vi "Data Analysis ver2.vi"() -> ()   [LabVIEW 2020]
uses:
  Data converted.ctl
  SignalConversion/FlattenedData.ctl
  Initialization/Param.ctl
  Initialization/ManualCtrl.ctl
  Initialization/DVESetting.ctl
  Initialization/CylinderCalibrNew.ctl
  SignalConversion/DAQChannelOffsets.ctl
  <vilib>/Analysis/Matrix/Datatypes/RealMatrix.ctl
  Data info.ctl
  Tasks/Task/Task.lvclass
  SignalConversion/ScaledData.ctl
  SignalConversion/Measrured TrapXYZ.ctl
  SignalConversion/Data Before Angle Compensation.ctl
  SignalConversion/Angle compensated data.ctl
  SignalConversion/XYZ Signals.ctl
  SignalConversion/Set TrapXYZ.ctl
  SignalConversion/DAQChannelRawData.ctl
  <vilib>/Utility/miscctls.llb/LVFontTypeDef.ctl
  <vilib>/Utility/file.llb/Read From Spreadsheet File (DBL).vi
  <vilib>/Utility/NIReport.llb/NI_report.lvclass
  SignalConversion/SignalConverson.lvlib
  Initialization/FileManagement/FileManagement.lvlib
  BasicVIs/BasicVIs.lvlib
  <vilib>/Analysis/NI_AALBase.lvlib
  <vilib>/Analysis/NI_AALPro.lvlib
  OldDAQtask/HeightFinder/HeightFinder.lvlib
  OldDAQtask/XYcenter/XYcenter.lvlib
  OldDAQtask/Measure angular gains/Measure angular gains.lvlib
  Initialization/Initialization.lvlib
  <vilib>/Analysis/Matrix/NI_Matrix.lvlib
panel:
  in  "stop":bool
  in  "Data Analysis Tab":T1(tab)
  in  "get description from raw data folder?":bool
  in  "Recalculate params":bool
  in  "Fit Method":u16(ring) items=["Reflective 1,3 order", "Symmetric 1,3 order", "1st and 3rd order Func Fit", "7thOrderExpandedWLC"]
  in  "Treat baseline parallel":bool=TRUE
  in  "FitMethod":u16(ring)=1 items=["Fit by two linear functions", "Fit by linear and quadratic "]
  out "%":i32(slide) max=35 scale=0.0..100.0
  in  "Apply new \"config.ini\" file":bool
  in  "configuration file path":path
  out "Trace #":i32(slide) max=35 scale=0.0..7.0
  in  "Raw data root folder":path
  in  "Start conversion":bool
  out "Task #":i32(slide) max=35 scale=0.0..20.0
  in  "Data info":T2 {"params array"."Cylinder Calibr"."ZsignalHeightDependence (1/nm)" format="%.4e"; "params array"."Instrument Calibr"."Psi" format="%#_2f"; "params array"."Manual Control"."Y peizo\n [nm]" step=100.0 scale=0.0..30000.0; "params array"."Manual Control"."AOM0 \nPower" scale=0.0..1.0; "params array"."Manual Control"."X piezo\n [nm]" step=100.0 scale=0.0..30000.0; "params array"."Manual Control"."Rotation Control"."mean freq  [MHz]\ndefault 39.99" min=0.0 step=0.01; "params array"."Manual Control"."Rotation Control"."B amp (0-120)" min=0.0 max=120.0 step=0.1 format="%.1f"; "params array"."Manual Control"."Rotation Control"."A amp (0-120)" min=0.0 max=120.0 step=0.1 format="%.1f"; "params array"."Manual Control"."Rotation Control"."Phase" scale=0.0..360.0; "params array"."Manual Control"."trap height\n [nm]" scale=1000.0..7500.0; "params array"."TaskIDs"."DAQ tasks"."Px taskID" format="%x"; "params array"."TaskIDs"."DAQ tasks"."Py taskID" format="%x"; "params array"."TaskIDs"."DAQ tasks"."Pz taskID" format="%x"; "params array"."TaskIDs"."DAQ tasks"."AOM taskID" format="%x"; "params array"."TaskIDs"."DAQ tasks"."Clock taskID" format="%x"; "params array"."TaskIDs"."DAQ tasks"."AI taskID" format="%x"}
  in  "key words in description":string
  out "Warning message":string
  out "Now converting file:":string
  out "pb1":dbl(slide) scale=0.0..1.0
  out "Descriptions of all traces":string="Trace_0000_Oscilloscope\\description: Initialization and oscilloscope data go here\r\nTrace_0014\\description: good 1\r\nTrace_0019\\description: good 2\r\nTrace_0037\\description: good 3\r\nTrace_0038\\description: good 4 braiding?\r\nTrace_0039\\description: good 4 braiding?\r\nTrace_0044\\description: good 5\r\nTrace_0049\\description: good 6-1\r\nTrace_0050\\description: good 6-2\r\nTrace_0053\\description: good 6-3 cannot achieve last step!!!\r\nTrace_0054\\description: error\r\nTrace_0058\\description: good 6-4 whole\r\nTrace_0059\\description: good 6-5 nucleosome depleted\r\nTrace_0060\\description: good 6-6 nucleosome depleted\r\nTrace_0061\\description: good 6-7 nucleosome depleted\r\nTrace_0062\\description: good 7 non-tc but stretching is good\r\nTrace_0067\\description: good ? 8\r\nTrace_0068\\description: good but break in the middle!\r\nTrace_0069\\description: good but break in the middle!\r\nTrace_0070\\description: braiding?\r\nTrace_0075\\description: good 9 1st multiple winding\r\nTrace_0082\\description: good but break in the middle 10\r\nTrace_0083\\description: good but break in the middle 11\r\nTrace_0086\\description: good weird?\r\nTrace_0092\\description: good only first trace sqeeze the nucleosome out\r\nTrace_0095\\description: good 12 only whole curve got\r\n"
  in  "Data (converted) to import":path
  out "Importing traces..":i32(slide) max=35 scale=0.0..1.0
  in  "Import converted data":bool
  out "Array 2":u32[][](array[colorbox])=[[10162682, 10293497, 10424313, 10555128, 10751479, 10947830, 11143925, 11405812, 11602162, 11864049, 12060399, 12322286, 12453100, 12649451, 12714986, 12780522, 12846058, 12780522, 12714986, 12649451, 12453100, 12322286, 12060399, 11864049, 11602162, 11405812, 11143925, 10947830, 10751479, 10555128, 10424313, 10293497], [10293497, 10424313, 10620664, 10817015, 11013110, 11274996, 11536627, 11864049, 12125679, 12453101, 12714987, 12976872, 13173479, 13369829, 13500900, 13566435, 13631970, 13566435, 13500900, 13369829, 13173479, 12976872, 12714987, 12453101, 12125679, 11864049, 11536627, 11274996, 11013110, 10817015, 10620664, 10424313], [10424313, 10620664, 10817015, 11078645, 11340276, 11667698, 11994864, 12387565, 12714986, 13107943, 13435364, 13762785, 13959390, 14221532, 14352602, 14418137, 14483673, 14418137, 14352602, 14221532, 13959390, 13762785, 13435364, 13107943, 12714986, 12387565, 11994864, 11667698, 11340276, 11078645, 10817015, 10620664], [10555128, 10817015, 11078645, 11405812, 11732978, 12125935, 12518636, 12976872, 13435365, 13828320, 14221532, 14549208, 14811348, 15073744, 15204814, 15270604, 15336139, 15270604, 15204814, 15073744, 14811348, 14549208, 14221532, 13828320, 13435365, 12976872, 12518636, 12125935, 11732978, 11405812, 11078645, 10817015], [10751479, 11013110, 11340276, 11732978, 12191215, 12649451, 13107943, 13631970, 14090461, 14549207, 15008209, 15336139, 15598534, 15795649, 15992510, 16058300, 16058299, 16058300, 15992510, 15795649, 15598534, 15336139, 15008209, 14549207, 14090461, 13631970, 13107943, 12649451, 12191215, 11732978, 11340276, 11013110], [10947830, 11274996, 11667698, 12125935, 12649451, 13173479, 13762785, 14287067, 14811348, 15270604, 15729860, 16058300, 16255669, 16453039, 16519082, 16585128, 16585383, 16585128, 16519082, 16453039, 16255669, 16058300, 15729860, 15270604, 14811348, 14287067, 13762785, 13173479, 12649451, 12125935, 11667698, 11274996], [11143925, 11536627, 11994864, 12518636, 13107943, 13762785, 14352602, 14942674, 15467465, 15926975, 16321204, 16519082, 16717217, 16718490, 16719508, 16720272, 16720527, 16720272, 16719508, 16718490, 16717217, 16519082, 16321204, 15926975, 15467465, 14942674, 14352602, 13762785, 13107943, 12518636, 11994864, 11536627], [11405812, 11864049, 12387565, 12976872, 13631970, 14287067, 14942674, 15532999, 16058300, 16453039, 16651426, 16718998, 16721291, 16657538, 16593531, 16529015, 16463733, 16529015, 16593531, 16657538, 16721291, 16718998, 16651426, 16453039, 16058300, 15532999, 14942674, 14287067, 13631970, 12976872, 12387565, 11864049], [11602162, 12125679, 12714986, 13435365, 14090461, 14811348, 15467465, 16058300, 16453293, 16717726, 16720527, 16657793, 16464244, 16139113, 15879009, 15683677, 15618395, 15683677, 15879009, 16139113, 16464244, 16657793, 16720527, 16717726, 16453293, 16058300, 15467465, 14811348, 14090461, 13435365, 12714986, 12125679], [11864049, 12453101, 13107943, 13828320, 14549207, 15270604, 15926975, 16453039, 16717726, 16721037, 16593531, 16204139, 15683677, 15162449, 14706249, 14445636, 14315074, 14445636, 14706249, 15162449, 15683677, 16204139, 16593531, 16721037, 16717726, 16453039, 15926975, 15270604, 14549207, 13828320, 13107943, 12453101], [12060399, 12714987, 13435364, 14221532, 15008209, 15729860, 16321204, 16651426, 16720527, 16593531, 16139368, 15423318, 14641223, 13858620, 13206067, 12814638, 12684077, 12814638, 13206067, 13858620, 14641223, 15423318, 16139368, 16593531, 16720527, 16651426, 16321204, 15729860, 15008209, 14221532, 13435364, 12714987], [12322286, 12976872, 13762785, 14549208, 15336139, 16058300, 16519082, 16718998, 16657793, 16204139, 15423318, 14445636, 13336629, 12357673, 11574306, 11052061, 10855964, 11052061, 11574306, 12357673, 13336629, 14445636, 15423318, 16204139, 16657793, 16718998, 16519082, 16058300, 15336139, 14549208, 13762785, 12976872], [12453100, 13173479, 13959390, 14811348, 15598534, 16255669, 16717217, 16721291, 16464244, 15683677, 14641223, 13336629, 12031270, 10855964, 9941781, 9353745, 9157904, 9353745, 9941781, 10855964, 12031270, 13336629, 14641223, 15683677, 16464244, 16721291, 16717217, 16255669, 15598534, 14811348, 13959390, 13173479], [12649451, 13369829, 14221532, 15073744, 15795649, 16453039, 16718490, 16657538, 16139113, 15162449, 13858620, 12357673, 10855964, 9549842, 8569868, 7916297, 7720456, 7916297, 8569868, 9549842, 10855964, 12357673, 13858620, 15162449, 16139113, 16657538, 16718490, 16453039, 15795649, 15073744, 14221532, 13369829], [12714986, 13500900, 14352602, 15204814, 15992510, 16519082, 16719508, 16593531, 15879009, 14706249, 13206067, 11574306, 9941781, 8569868, 7524359, 6870789, 6609156, 6870789, 7524359, 8569868, 9941781, 11574306, 13206067, 14706249, 15879009, 16593531, 16719508, 16519082, 15992510, 15204814, 14352602, 13500900], [12780522, 13566435, 14418137, 15270604, 16058300, 16585128, 16720272, 16529015, 15683677, 14445636, 12814638, 11052061, 9353745, 7916297, 6870789, 6216963, 5955586, 6216963, 6870789, 7916297, 9353745, 11052061, 12814638, 14445636, 15683677, 16529015, 16720272, 16585128, 16058300, 15270604, 14418137, 13566435], [12846058, 13631970, 14483673, 15336139, 16058299, 16585383, 16720527, 16463733, 15618395, 14315074, 12684077, 10855964, 9157904, 7720456, 6609156, 5955586, 5759490, 5955586, 6609156, 7720456, 9157904, 10855964, 12684077, 14315074, 15618395, 16463733, 16720527, 16585383, 16058299, 15336139, 14483673, 13631970], [12780522, 13566435, 14418137, 15270604, 16058300, 16585128, 16720272, 16529015, 15683677, 14445636, 12814638, 11052061, 9353745, 7916297, 6870789, 6216963, 5955586, 6216963, 6870789, 7916297, 9353745, 11052061, 12814638, 14445636, 15683677, 16529015, 16720272, 16585128, 16058300, 15270604, 14418137, 13566435], [12714986, 13500900, 14352602, 15204814, 15992510, 16519082, 16719508, 16593531, 15879009, 14706249, 13206067, 11574306, 9941781, 8569868, 7524359, 6870789, 6609156, 6870789, 7524359, 8569868, 9941781, 11574306, 13206067, 14706249, 15879009, 16593531, 16719508, 16519082, 15992510, 15204814, 14352602, 13500900], [12649451, 13369829, 14221532, 15073744, 15795649, 16453039, 16718490, 16657538, 16139113, 15162449, 13858620, 12357673, 10855964, 9549842, 8569868, 7916297, 7720456, 7916297, 8569868, 9549842, 10855964, 12357673, 13858620, 15162449, 16139113, 16657538, 16718490, 16453039, 15795649, 15073744, 14221532, 13369829], [12453100, 13173479, 13959390, 14811348, 15598534, 16255669, 16717217, 16721291, 16464244, 15683677, 14641223, 13336629, 12031270, 10855964, 9941781, 9353745, 9157904, 9353745, 9941781, 10855964, 12031270, 13336629, 14641223, 15683677, 16464244, 16721291, 16717217, 16255669, 15598534, 14811348, 13959390, 13173479], [12322286, 12976872, 13762785, 14549208, 15336139, 16058300, 16519082, 16718998, 16657793, 16204139, 15423318, 14445636, 13336629, 12357673, 11574306, 11052061, 10855964, 11052061, 11574306, 12357673, 13336629, 14445636, 15423318, 16204139, 16657793, 16718998, 16519082, 16058300, 15336139, 14549208, 13762785, 12976872], [12060399, 12714987, 13435364, 14221532, 15008209, 15729860, 16321204, 16651426, 16720527, 16593531, 16139368, 15423318, 14641223, 13858620, 13206067, 12814638, 12684077, 12814638, 13206067, 13858620, 14641223, 15423318, 16139368, 16593531, 16720527, 16651426, 16321204, 15729860, 15008209, 14221532, 13435364, 12714987], [11864049, 12453101, 13107943, 13828320, 14549207, 15270604, 15926975, 16453039, 16717726, 16721037, 16593531, 16204139, 15683677, 15162449, 14706249, 14445636, 14315074, 14445636, 14706249, 15162449, 15683677, 16204139, 16593531, 16721037, 16717726, 16453039, 15926975, 15270604, 14549207, 13828320, 13107943, 12453101], [11602162, 12125679, 12714986, 13435365, 14090461, 14811348, 15467465, 16058300, 16453293, 16717726, 16720527, 16657793, 16464244, 16139113, 15879009, 15683677, 15618395, 15683677, 15879009, 16139113, 16464244, 16657793, 16720527, 16717726, 16453293, 16058300, 15467465, 14811348, 14090461, 13435365, 12714986, 12125679], [11405812, 11864049, 12387565, 12976872, 13631970, 14287067, 14942674, 15532999, 16058300, 16453039, 16651426, 16718998, 16721291, 16657538, 16593531, 16529015, 16463733, 16529015, 16593531, 16657538, 16721291, 16718998, 16651426, 16453039, 16058300, 15532999, 14942674, 14287067, 13631970, 12976872, 12387565, 11864049], [11143925, 11536627, 11994864, 12518636, 13107943, 13762785, 14352602, 14942674, 15467465, 15926975, 16321204, 16519082, 16717217, 16718490, 16719508, 16720272, 16720527, 16720272, 16719508, 16718490, 16717217, 16519082, 16321204, 15926975, 15467465, 14942674, 14352602, 13762785, 13107943, 12518636, 11994864, 11536627], [10947830, 11274996, 11667698, 12125935, 12649451, 13173479, 13762785, 14287067, 14811348, 15270604, 15729860, 16058300, 16255669, 16453039, 16519082, 16585128, 16585383, 16585128, 16519082, 16453039, 16255669, 16058300, 15729860, 15270604, 14811348, 14287067, 13762785, 13173479, 12649451, 12125935, 11667698, 11274996], [10751479, 11013110, 11340276, 11732978, 12191215, 12649451, 13107943, 13631970, 14090461, 14549207, 15008209, 15336139, 15598534, 15795649, 15992510, 16058300, 16058299, 16058300, 15992510, 15795649, 15598534, 15336139, 15008209, 14549207, 14090461, 13631970, 13107943, 12649451, 12191215, 11732978, 11340276, 11013110], [10555128, 10817015, 11078645, 11405812, 11732978, 12125935, 12518636, 12976872, 13435365, 13828320, 14221532, 14549208, 14811348, 15073744, 15204814, 15270604, 15336139, 15270604, 15204814, 15073744, 14811348, 14549208, 14221532, 13828320, 13435365, 12976872, 12518636, 12125935, 11732978, 11405812, 11078645, 10817015], [10424313, 10620664, 10817015, 11078645, 11340276, 11667698, 11994864, 12387565, 12714986, 13107943, 13435364, 13762785, 13959390, 14221532, 14352602, 14418137, 14483673, 14418137, 14352602, 14221532, 13959390, 13762785, 13435364, 13107943, 12714986, 12387565, 11994864, 11667698, 11340276, 11078645, 10817015, 10620664], [10293497, 10424313, 10620664, 10817015, 11013110, 11274996, 11536627, 11864049, 12125679, 12453101, 12714987, 12976872, 13173479, 13369829, 13500900, 13566435, 13631970, 13566435, 13500900, 13369829, 13173479, 12976872, 12714987, 12453101, 12125679, 11864049, 11536627, 11274996, 11013110, 10817015, 10620664, 10424313]]
  out "Fitting result (see block diagram the meanings)":T9
  in  "fit option":u16(ring) items=["Do nothing", "Linear fit", "EWLC fit", "Hat curve fit"]
  out "XY Graph":T10(graph)
  in  "All tasks in tasklist":i32[](listbox)
  in  "Y Axis to plot":i32(ring)=12 items=["V_A' [V]", "V_D' [V]", "V_P'  [V]", "V_S' [V]", "V_L' [V]", "V_R' [V]", "V_sum' [V]", "V_x [V]", "V_y [V]", "V_px' [V]", "V_py' [V]", "V_pz' [V]", "dt [s]", "Vpx_AO [V]", "Vpy_AO [V]", "Vpz_AO [V]", "scan backlog", "LockInPhase", "TrapX [nm]", "TrapY [nm]", "TrapZ [nm]", "V_A [V]", "V_D [V]", "V_P [V]", "V_S [V]", "V_L [V]", "V_R [V]", "V_sum [V]", "V_x [V]", "V_y [V]", "P power [mW]", "S power [mW]", "angle compensated P power [W]", "angle compensated S power [W]", "angle compensated V_L", "angle compensated V_R", "angle compensated V_sum [V]", "angle compensated V_x [V]", "angle compensated V_y [V]", "Psi [rad]", "Laser power before objective[W]", "E_in", "E_out", "Delta E", "X signal", "Y signal", "Z signal", "TrapX (AO) [nm]", "TrapY (AO) [nm]", "TrapZ (AO) [nm]", "Fz [pN]", "Zext [nm]", "Tau [pNnm]", "Turn", "Fx [pN]", "Xext [nm]", "Fy [pN]", "Yext [nm]", "time [s]", "Delta Z signal", "Delta Z bead [nm]", "Z bead [nm]", "Delta TrapZ [nm]", "Delta Xsignal", "X bead [nm]", "Delta Ysignal", "Y bead [nm]", "Stop Condition"]
  in  "X Axis to plot":i32(ring)=12 items=["V_A' [V]", "V_D' [V]", "V_P'  [V]", "V_S' [V]", "V_L' [V]", "V_R' [V]", "V_sum' [V]", "V_x [V]", "V_y [V]", "V_px' [V]", "V_py' [V]", "V_pz' [V]", "dt [s]", "Vpx_AO [V]", "Vpy_AO [V]", "Vpz_AO [V]", "scan backlog", "LockInPhase", "TrapX [nm]", "TrapY [nm]", "TrapZ [nm]", "V_A [V]", "V_D [V]", "V_P [V]", "V_S [V]", "V_L [V]", "V_R [V]", "V_sum [V]", "V_x [V]", "V_y [V]", "P power [mW]", "S power [mW]", "angle compensated P power [W]", "angle compensated S power [W]", "angle compensated V_L", "angle compensated V_R", "angle compensated V_sum [V]", "angle compensated V_x [V]", "angle compensated V_y [V]", "Psi [rad]", "Laser power before objective[W]", "E_in", "E_out", "Delta E", "X signal", "Y signal", "Z signal", "TrapX (AO) [nm]", "TrapY (AO) [nm]", "TrapZ (AO) [nm]", "Fz [pN]", "Zext [nm]", "Tau [pNnm]", "Turn", "Fx [pN]", "Xext [nm]", "Fy [pN]", "Yext [nm]", "time [s]", "Delta Z signal", "Delta Z bead [nm]", "Z bead [nm]", "Delta TrapZ [nm]", "Delta Xsignal", "X bead [nm]", "Delta Ysignal", "Y bead [nm]", "Stop Condition"]
  in  "All traces":i32(listbox)
  in  "Delete trace":bool
  in  "Undo delete":bool
  out "Histogram Graph Y signal (the upmost task)":T11(graph)
  out "mean":dbl format="%0.2f"
  out "s.d.":dbl format="%0.2f"
  out "sigma":dbl format="%0.2f"
  out "center":dbl format="%0.2f"
  in  "Fit":bool
  in  "save to txt":bool
  in  "Save graph":bool
  out "Laser power [W]":dbl format="%0.2f"
  out "Laser power fluctuation [W]":dbl format="%0.2f"
  out "Description":string
  in  "Tab Control":T12(tab)=enum."Settings"
  out "XY Graph for plot 1":T10(graph)
  out "XY Graph for plot 2":T10(graph)
  in  "X Axis to plot 2":i32(ring)=12 items=["V_A' [V]", "V_D' [V]", "V_P'  [V]", "V_S' [V]", "V_L' [V]", "V_R' [V]", "V_sum' [V]", "V_x [V]", "V_y [V]", "V_px' [V]", "V_py' [V]", "V_pz' [V]", "dt [s]", "Vpx_AO [V]", "Vpy_AO [V]", "Vpz_AO [V]", "scan backlog", "LockInPhase", "TrapX [nm]", "TrapY [nm]", "TrapZ [nm]", "V_A [V]", "V_D [V]", "V_P [V]", "V_S [V]", "V_L [V]", "V_R [V]", "V_sum [V]", "V_x [V]", "V_y [V]", "P power [mW]", "S power [mW]", "angle compensated P power [W]", "angle compensated S power [W]", "angle compensated V_L", "angle compensated V_R", "angle compensated V_sum [V]", "angle compensated V_x [V]", "angle compensated V_y [V]", "Psi [rad]", "Laser power before objective[W]", "E_in", "E_out", "Delta E", "X signal", "Y signal", "Z signal", "TrapX (AO) [nm]", "TrapY (AO) [nm]", "TrapZ (AO) [nm]", "Fz [pN]", "Zext [nm]", "Tau [pNnm]", "Turn", "Fx [pN]", "Xext [nm]", "Fy [pN]", "Yext [nm]", "time [s]", "Delta Z signal", "Delta Z bead [nm]", "Z bead [nm]", "Delta TrapZ [nm]", "Delta Xsignal", "X bead [nm]", "Delta Ysignal", "Y bead [nm]", "Stop Condition"]
  in  "Y Axis to plot 2":i32(ring)=12 items=["V_A' [V]", "V_D' [V]", "V_P'  [V]", "V_S' [V]", "V_L' [V]", "V_R' [V]", "V_sum' [V]", "V_x [V]", "V_y [V]", "V_px' [V]", "V_py' [V]", "V_pz' [V]", "dt [s]", "Vpx_AO [V]", "Vpy_AO [V]", "Vpz_AO [V]", "scan backlog", "LockInPhase", "TrapX [nm]", "TrapY [nm]", "TrapZ [nm]", "V_A [V]", "V_D [V]", "V_P [V]", "V_S [V]", "V_L [V]", "V_R [V]", "V_sum [V]", "V_x [V]", "V_y [V]", "P power [mW]", "S power [mW]", "angle compensated P power [W]", "angle compensated S power [W]", "angle compensated V_L", "angle compensated V_R", "angle compensated V_sum [V]", "angle compensated V_x [V]", "angle compensated V_y [V]", "Psi [rad]", "Laser power before objective[W]", "E_in", "E_out", "Delta E", "X signal", "Y signal", "Z signal", "TrapX (AO) [nm]", "TrapY (AO) [nm]", "TrapZ (AO) [nm]", "Fz [pN]", "Zext [nm]", "Tau [pNnm]", "Turn", "Fx [pN]", "Xext [nm]", "Fy [pN]", "Yext [nm]", "time [s]", "Delta Z signal", "Delta Z bead [nm]", "Z bead [nm]", "Delta TrapZ [nm]", "Delta Xsignal", "X bead [nm]", "Delta Ysignal", "Y bead [nm]", "Stop Condition"]
  in  "Plot 1 Options":T14={"Color"=[0, 16711680, 6618880, 16860, 16750610, 4390878, 8388847, 16775234, 5878015, 16740807], "X axis label"="example x", "Y axis label"="example y", "BG color"=16776176, "% axis off"=0.1, "% margin "=2.0, "F: JPEG\nT: PNG"=TRUE, "Font"={"Font Name"="Times New Roman", "Size"=40, "Bold"=TRUE, "Italic"=FALSE, "Underline"=FALSE, "Strikeout"=FALSE, "Color"=0}, "Plot Line Width"=2, "X format str"="%.0f", "Y format str"="%.0f", "axis range"={"Max X scale"=0.0, "Min X scale"=0.0, "Max Y scale"=0.0, "Min Y scale"=0.0}, "auto scale?"=TRUE}
  in  "Plot 2 Options":T14={"Color"=[0, 16711680, 6618880, 16860, 16750610, 4390878, 8388847, 16775234, 5878015, 16740807], "X axis label"="example x", "Y axis label"="example y", "BG color"=16776176, "% axis off"=0.1, "% margin "=2.0, "F: JPEG\nT: PNG"=TRUE, "Font"={"Font Name"="Times New Roman", "Size"=40, "Bold"=TRUE, "Italic"=FALSE, "Underline"=FALSE, "Strikeout"=FALSE, "Color"=0}, "Plot Line Width"=2, "X format str"="%.2f", "Y format str"="%.2f", "axis range"={"Max X scale"=0.0, "Min X scale"=0.0, "Max Y scale"=0.0, "Min Y scale"=0.0}, "auto scale?"=TRUE}
  in  "CreateReport":bool
  in  "Max digit of index":i32=4
  in  "Key words":string="Trace_"
  in  "refresh trace list":bool
  out "array delete order":i32[](array[numeric])
  out "All trace  info":T15(array[cluster]) caption="Folder name                    Description                                                                              Folder index     Key words           Log in finding index"
  in  "path":path caption="path txt saving path"
  out "All descriptions":string="Trace_0000_Oscilloscope\\description: Initialization and oscilloscope data go here\r\nTrace_0014\\description: good 1\r\nTrace_0019\\description: good 2\r\nTrace_0037\\description: good 3\r\nTrace_0038\\description: good 4 braiding?\r\nTrace_0039\\description: good 4 braiding?\r\nTrace_0044\\description: good 5\r\nTrace_0049\\description: good 6-1\r\nTrace_0050\\description: good 6-2\r\nTrace_0053\\description: good 6-3 cannot achieve last step!!!\r\nTrace_0054\\description: error\r\nTrace_0058\\description: good 6-4 whole\r\nTrace_0059\\description: good 6-5 nucleosome depleted\r\nTrace_0060\\description: good 6-6 nucleosome depleted\r\nTrace_0061\\description: good 6-7 nucleosome depleted\r\nTrace_0062\\description: good 7 non-tc but stretching is good\r\nTrace_0067\\description: good ? 8\r\nTrace_0068\\description: good but break in the middle!\r\nTrace_0069\\description: good but break in the middle!\r\nTrace_0070\\description: braiding?\r\nTrace_0075\\description: good 9 1st multiple winding\r\nTrace_0082\\description: good but break in the middle 10\r\nTrace_0083\\description: good but break in the middle 11\r\nTrace_0086\\description: good weird?\r\nTrace_0092\\description: good only first trace sqeeze the nucleosome out\r\nTrace_0095\\description: good 12 only whole curve got\r\n"
  in  "Graph autoname":string[](array[string])
  out "Array of Params out":T3[](array[typedef]) {"Cylinder Calibr"."ZsignalHeightDependence (1/nm)" format="%.4e"; "Instrument Calibr"."Psi" format="%#_2f"; "Manual Control"."Y peizo\n [nm]" step=100.0 scale=0.0..30000.0; "Manual Control"."AOM0 \nPower" scale=0.0..1.0; "Manual Control"."X piezo\n [nm]" step=100.0 scale=0.0..30000.0; "Manual Control"."Rotation Control"."mean freq  [MHz]\ndefault 39.99" min=0.0 step=0.01; "Manual Control"."Rotation Control"."B amp (0-120)" min=0.0 max=120.0 step=0.1 format="%.1f"; "Manual Control"."Rotation Control"."A amp (0-120)" min=0.0 max=120.0 step=0.1 format="%.1f"; "Manual Control"."Rotation Control"."Phase" scale=0.0..360.0; "Manual Control"."trap height\n [nm]" scale=1000.0..7500.0; "TaskIDs"."DAQ tasks"."Px taskID" format="%x"; "TaskIDs"."DAQ tasks"."Py taskID" format="%x"; "TaskIDs"."DAQ tasks"."Pz taskID" format="%x"; "TaskIDs"."DAQ tasks"."AOM taskID" format="%x"; "TaskIDs"."DAQ tasks"."Clock taskID" format="%x"; "TaskIDs"."DAQ tasks"."AI taskID" format="%x"}
  in  "Array of Params const":T3[](array[typedef]) {"Cylinder Calibr"."ZsignalHeightDependence (1/nm)" format="%.4e"; "Instrument Calibr"."Psi" format="%#_2f"; "Manual Control"."Y peizo\n [nm]" step=100.0 scale=0.0..30000.0; "Manual Control"."AOM0 \nPower" scale=0.0..1.0; "Manual Control"."X piezo\n [nm]" step=100.0 scale=0.0..30000.0; "Manual Control"."Rotation Control"."mean freq  [MHz]\ndefault 39.99" min=0.0 step=0.01; "Manual Control"."Rotation Control"."B amp (0-120)" min=0.0 max=120.0 step=0.1 format="%.1f"; "Manual Control"."Rotation Control"."A amp (0-120)" min=0.0 max=120.0 step=0.1 format="%.1f"; "Manual Control"."Rotation Control"."Phase" scale=0.0..360.0; "Manual Control"."trap height\n [nm]" scale=1000.0..7500.0; "TaskIDs"."DAQ tasks"."Px taskID" format="%x"; "TaskIDs"."DAQ tasks"."Py taskID" format="%x"; "TaskIDs"."DAQ tasks"."Pz taskID" format="%x"; "TaskIDs"."DAQ tasks"."AOM taskID" format="%x"; "TaskIDs"."DAQ tasks"."Clock taskID" format="%x"; "TaskIDs"."DAQ tasks"."AI taskID" format="%x"}
  in  "All data after scaling":T16
  in  "All DAQ channels":T22
  in  "empty data info":T2 {"params array"."Cylinder Calibr"."ZsignalHeightDependence (1/nm)" format="%.4e"; "params array"."Instrument Calibr"."Psi" format="%#_2f"; "params array"."Manual Control"."Y peizo\n [nm]" step=100.0 scale=0.0..30000.0; "params array"."Manual Control"."AOM0 \nPower" scale=0.0..1.0; "params array"."Manual Control"."X piezo\n [nm]" step=100.0 scale=0.0..30000.0; "params array"."Manual Control"."Rotation Control"."mean freq  [MHz]\ndefault 39.99" min=0.0 step=0.01; "params array"."Manual Control"."Rotation Control"."B amp (0-120)" min=0.0 max=120.0 step=0.1 format="%.1f"; "params array"."Manual Control"."Rotation Control"."A amp (0-120)" min=0.0 max=120.0 step=0.1 format="%.1f"; "params array"."Manual Control"."Rotation Control"."Phase" scale=0.0..360.0; "params array"."Manual Control"."trap height\n [nm]" scale=1000.0..7500.0; "params array"."TaskIDs"."DAQ tasks"."Px taskID" format="%x"; "params array"."TaskIDs"."DAQ tasks"."Py taskID" format="%x"; "params array"."TaskIDs"."DAQ tasks"."Pz taskID" format="%x"; "params array"."TaskIDs"."DAQ tasks"."AOM taskID" format="%x"; "params array"."TaskIDs"."DAQ tasks"."Clock taskID" format="%x"; "params array"."TaskIDs"."DAQ tasks"."AI taskID" format="%x"}
  out "~All data converted":T23 {"Array of Params"."Cylinder Calibr"."ZsignalHeightDependence (1/nm)" format="%.4e"; "Array of Params"."Instrument Calibr"."Psi" format="%#_2f"; "Array of Params"."Manual Control"."Y peizo\n [nm]" step=100.0 scale=0.0..30000.0; "Array of Params"."Manual Control"."AOM0 \nPower" scale=0.0..1.0; "Array of Params"."Manual Control"."X piezo\n [nm]" step=100.0 scale=0.0..30000.0; "Array of Params"."Manual Control"."Rotation Control"."mean freq  [MHz]\ndefault 39.99" min=0.0 step=0.01; "Array of Params"."Manual Control"."Rotation Control"."B amp (0-120)" min=0.0 max=120.0 step=0.1 format="%.1f"; "Array of Params"."Manual Control"."Rotation Control"."A amp (0-120)" min=0.0 max=120.0 step=0.1 format="%.1f"; "Array of Params"."Manual Control"."Rotation Control"."Phase" scale=0.0..360.0; "Array of Params"."Manual Control"."trap height\n [nm]" scale=1000.0..7500.0; "Array of Params"."TaskIDs"."DAQ tasks"."Px taskID" format="%x"; "Array of Params"."TaskIDs"."DAQ tasks"."Py taskID" format="%x"; "Array of Params"."TaskIDs"."DAQ tasks"."Pz taskID" format="%x"; "Array of Params"."TaskIDs"."DAQ tasks"."AOM taskID" format="%x"; "Array of Params"."TaskIDs"."DAQ tasks"."Clock taskID" format="%x"; "Array of Params"."TaskIDs"."DAQ tasks"."AI taskID" format="%x"}
  out "data deleted":T23 {"Array of Params"."Cylinder Calibr"."ZsignalHeightDependence (1/nm)" format="%.4e"; "Array of Params"."Instrument Calibr"."Psi" format="%#_2f"; "Array of Params"."Manual Control"."Y peizo\n [nm]" step=100.0 scale=0.0..30000.0; "Array of Params"."Manual Control"."AOM0 \nPower" scale=0.0..1.0; "Array of Params"."Manual Control"."X piezo\n [nm]" step=100.0 scale=0.0..30000.0; "Array of Params"."Manual Control"."Rotation Control"."mean freq  [MHz]\ndefault 39.99" min=0.0 step=0.01; "Array of Params"."Manual Control"."Rotation Control"."B amp (0-120)" min=0.0 max=120.0 step=0.1 format="%.1f"; "Array of Params"."Manual Control"."Rotation Control"."A amp (0-120)" min=0.0 max=120.0 step=0.1 format="%.1f"; "Array of Params"."Manual Control"."Rotation Control"."Phase" scale=0.0..360.0; "Array of Params"."Manual Control"."trap height\n [nm]" scale=1000.0..7500.0; "Array of Params"."TaskIDs"."DAQ tasks"."Px taskID" format="%x"; "Array of Params"."TaskIDs"."DAQ tasks"."Py taskID" format="%x"; "Array of Params"."TaskIDs"."DAQ tasks"."Pz taskID" format="%x"; "Array of Params"."TaskIDs"."DAQ tasks"."AOM taskID" format="%x"; "Array of Params"."TaskIDs"."DAQ tasks"."Clock taskID" format="%x"; "Array of Params"."TaskIDs"."DAQ tasks"."AI taskID" format="%x"}
  in  "data of tasks in single trace":T25
  in  "empty data converted":T23 {"Array of Params"."Cylinder Calibr"."ZsignalHeightDependence (1/nm)" format="%.4e"; "Array of Params"."Instrument Calibr"."Psi" format="%#_2f"; "Array of Params"."Manual Control"."Y peizo\n [nm]" step=100.0 scale=0.0..30000.0; "Array of Params"."Manual Control"."AOM0 \nPower" scale=0.0..1.0; "Array of Params"."Manual Control"."X piezo\n [nm]" step=100.0 scale=0.0..30000.0; "Array of Params"."Manual Control"."Rotation Control"."mean freq  [MHz]\ndefault 39.99" min=0.0 step=0.01; "Array of Params"."Manual Control"."Rotation Control"."B amp (0-120)" min=0.0 max=120.0 step=0.1 format="%.1f"; "Array of Params"."Manual Control"."Rotation Control"."A amp (0-120)" min=0.0 max=120.0 step=0.1 format="%.1f"; "Array of Params"."Manual Control"."Rotation Control"."Phase" scale=0.0..360.0; "Array of Params"."Manual Control"."trap height\n [nm]" scale=1000.0..7500.0; "Array of Params"."TaskIDs"."DAQ tasks"."Px taskID" format="%x"; "Array of Params"."TaskIDs"."DAQ tasks"."Py taskID" format="%x"; "Array of Params"."TaskIDs"."DAQ tasks"."Pz taskID" format="%x"; "Array of Params"."TaskIDs"."DAQ tasks"."AOM taskID" format="%x"; "Array of Params"."TaskIDs"."DAQ tasks"."Clock taskID" format="%x"; "Array of Params"."TaskIDs"."DAQ tasks"."AI taskID" format="%x"}
  # "Tools"
  # "Statistics:"
  # "Channels in page 2:"
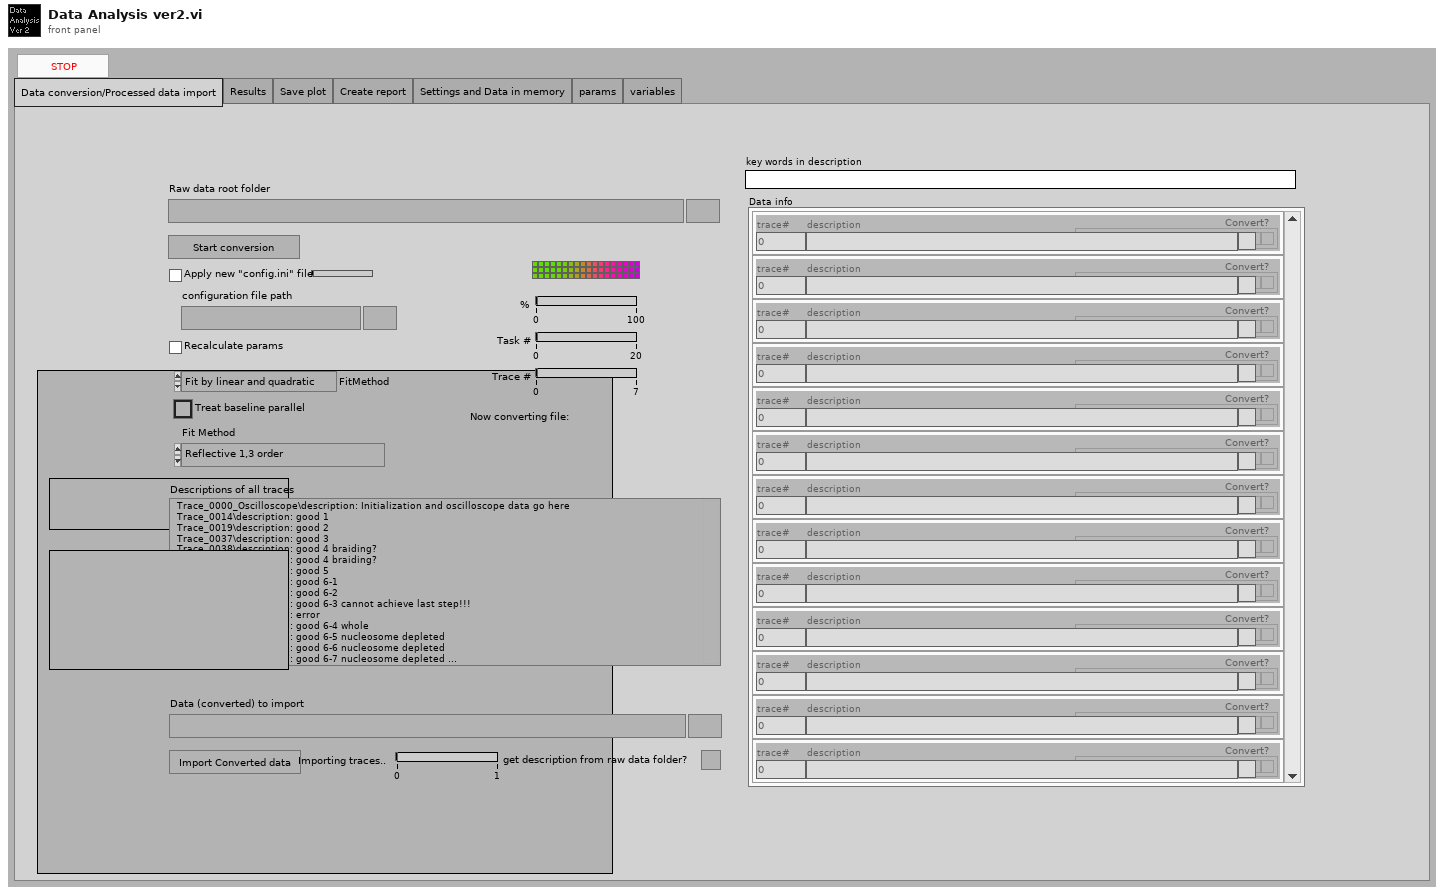
[diagram p1: front panel]
types:
  T1 = enum32{"Data conversion/Processed data import", "Results", "Save plot", "Create report", "Settings and Data in memory", "params", "variables"}
  T2 = typedef "Data info.ctl" = cluster{"trace#":i32, cluster{"index":i32, "File path":path, "File name":string}[], "description":string, "Convert?":bool, "params array":T3[], "Array":refnum<class "Task.lvclass">[]}[]
  T3 = typedef "Initialization.lvlib/Param.ctl" = cluster{"TaskIDs":cluster{"DAQ tasks":cluster{"Px taskID":u32, "Py taskID":u32, "Pz taskID":u32, "AOM taskID":u32, "Clock taskID":u32, "AI taskID":u32}, "DVEHandle":refnum<file>}, "Manual Control":T4, "Piezo Calibr":cluster{"Px2Vx(AO)":dbl, "Py2Vy(AO)":dbl, "Pz2Vz(AO)":dbl, "Min Px":dbl, "Min Py":dbl, "Min Pz":dbl, "Max Px":dbl, "Max Py":dbl, "Max Pz":dbl, "Vx0 (V)":dbl, "Vy0 (V)":dbl, "Vz0 (V)":dbl}, "Instrument Calibr":cluster{"Angular compensation coeffs":dbl[][], "TetherCenter":cluster{"TrapX_AO 0 [nm]":dbl, "TrapY_AO 0 [nm]":dbl, "TrapZ_AO 0 [nm]":dbl}, "XYZsignal baseline":cluster{"Xsignal0":dbl, "Ysignal0":dbl, "Zsignal0":dbl, "Zsig slope":dbl, "Z bead0":dbl}, "S and P to Vs0":cluster{"Vs0/P":dbl, "Vs0/S":dbl}, "Psi":dbl, "ePS:eRL drift correlation":cluster{"Interc P":dbl, "Slope P":dbl, "Interc S":dbl, "Slope S":dbl}, "Current piezo volt AO":cluster{"Vpx_AO [V]":dbl, "Vpy_AO [V]":dbl, "Vpz_AO [V]":dbl}}, "Cylinder Calibr":T6, "DAQParams":cluster{"Buffer size":dbl, "Scanning rate":dbl, "Average":dbl, "Sampling rate":dbl, "set dt":dbl}, "DAQ channel offsets":T7, "Z bead polynomial coeffs":dbl[], "Skip button ref":refnum<vi>, "z bead lookup table":cluster{"z signal":dbl[], "z bead":dbl[]}, "SP->power Matrix":T8, "Ms2p":T8, "Mp2s":T8, "Polynomial coeff V_px,y,z 2 position (nm)":dbl[][]}
  T4 = typedef "Initialization.lvlib/ManualCtrl.ctl" = cluster{"Rotation Control":T5, "X piezo\n [nm]":dbl, "Y peizo\n [nm]":dbl, "trap height\n [nm]":dbl, "AOM0 \nPower":dbl}
  T5 = typedef "Initialization.lvlib/DVESetting.ctl" = cluster{"Phase":dbl, "A amp (0-120)":dbl, "B amp (0-120)":dbl, "mean freq  [MHz]\ndefault 39.99":dbl, "freq difference [Hz]":dbl, "Enable A":bool, "Enable B":bool}
  T6 = typedef "Initialization.lvlib/CylinderCalibrNew.ctl" = cluster{"ZStiff":dbl, "Zsens":dbl, "AngStiff":dbl, "XStiff":dbl, "Xsens":dbl, "MaxEllip":dbl, "YStiff":dbl, "Ysens":dbl, "FocalShift":dbl, "Sfz":dbl, "1/Sz":dbl, "Stau":dbl, "Sfx":dbl, "1/Sx":dbl, "1/Sang":dbl, "Sfy":dbl, "1/Sy":dbl, "1/focal":dbl, "ZsignalHeightDependence (1/nm)":dbl}
  T7 = typedef "SignalConverson.lvlib/DAQChannelOffsets.ctl" = cluster{"A0 [V]":dbl, "D0 [V]":dbl, "P0  [V]":dbl, "S0 [V]":dbl, "L0 [V]":dbl, "R0 [V]":dbl, "Vpx0 [V]":dbl, "Vpy0 [V]":dbl, "Vpz0 [V]":dbl, "Vsum0 [V]":dbl, "Vpx_AO0 [V]":dbl, "Vpy_AO0 [V]":dbl, "Vpz_AO0 [V]":dbl}
  T8 = typedef "NI_Matrix.lvlib/RealMatrix.ctl" = dbl[][]
  T9 = cluster{"coeff 0":dbl, "coeff 1":dbl, "coeff 2":dbl, "coeff 3":dbl}
  T10 = cluster{"Processed data":dbl[], "Processed data":dbl[]}[]
  T11 = cluster{"X Values":dbl[], "Best Gaussian Fit":dbl[]}[]
  T12 = enum32{"Plot 1 (=plot in \"Reults\" tab)", "Page 2", "Settings"}
  T13 = typedef "LVFontTypeDef.ctl" = cluster{"Font Name":string, "Size":u16, "Bold":bool, "Italic":bool, "Underline":bool, "Strikeout":bool, "Color":u32}
  T14 = cluster{"Color":u32[], "X axis label":string, "Y axis label":string, "BG color":u32, "% axis off":dbl, "% margin ":dbl, "F: JPEG\nT: PNG":bool, "Font":T13, "Plot Line Width":u8, "X format str":string, "Y format str":string, "axis range":cluster{"Max X scale":dbl, "Min X scale":dbl, "Max Y scale":dbl, "Min Y scale":dbl}, "auto scale?":bool}
  T15 = cluster{"Folder index":i32, "Date modefied":i32, "Folder name":string, "Description":string, "Key words":string, "Log in Finding index":string}[]
  T16 = typedef "SignalConverson.lvlib/ScaledData.ctl" = cluster{"Measured TrapXYZ":T17, "Data before ang comp":T18, "Data after angle compensation":T19, "X,Y,Z signal":T20, "Set TrapXYZ":T21}
  T17 = typedef "SignalConverson.lvlib/Measrured TrapXYZ.ctl" = cluster{"TrapX [nm]":dbl, "TrapY [nm]":dbl, "TrapZ [nm]":dbl}
  T18 = typedef "SignalConverson.lvlib/Data Before Angle Compensation.ctl" = cluster{"V_A [V]":dbl, "V_D [V]":dbl, "V_P [V]":dbl, "V_S [V]":dbl, "V_L [V]":dbl, "V_R [V]":dbl, "V_sum [V]":dbl, "V_x [V]":dbl, "V_y [V]":dbl, "P power [mW]":dbl, "S power [mW]":dbl}
  T19 = typedef "SignalConverson.lvlib/Angle compensated data.ctl" = cluster{"angle compensated P power [W]":dbl, "angle compensated S power [W]":dbl, "angle compensated V_L":dbl, "angle compensated V_R":dbl, "angle compensated V_sum [V]":dbl, "angle compensated V_x [V]":dbl, "angle compensated V_y [V]":dbl, "Psi [rad]":dbl, "Laser power before objective[W]":dbl, "E_in":dbl, "E_out":dbl, "Delta E":dbl}
  T20 = typedef "SignalConverson.lvlib/XYZ Signals.ctl" = cluster{"X signal":dbl, "Y signal":dbl, "Z signal":dbl}
  T21 = typedef "SignalConverson.lvlib/Set TrapXYZ.ctl" = cluster{"TrapX (AO) [nm]":dbl, "TrapY (AO) [nm]":dbl, "TrapZ (AO) [nm]":dbl}
  T22 = typedef "SignalConverson.lvlib/DAQChannelRawData.ctl" = cluster{"V_A' [V]":dbl, "V_D' [V]":dbl, "V_P'  [V]":dbl, "V_S' [V]":dbl, "V_L' [V]":dbl, "V_R' [V]":dbl, "V_sum' [V]":dbl, "V_x [V]":dbl, "V_y [V]":dbl, "V_px' [V]":dbl, "V_py' [V]":dbl, "V_pz' [V]":dbl, "dt [s]":dbl, "Vpx_AO [V]":dbl, "Vpy_AO [V]":dbl, "Vpz_AO [V]":dbl, "scan backlog":u32, "LockInPhase":dbl}
  T23 = typedef "Data converted.ctl" = cluster{cluster{"trace (folder) name":string, "task (file) name":string, "processed data":T24[]}[], "tasklist (name)":string[], "trace name":string, "description":string, "Array of Params":T3[]}[]
  T24 = typedef "SignalConverson.lvlib/FlattenedData.ctl" = cluster{"V_A' [V]":dbl, "V_D' [V]":dbl, "V_P'  [V]":dbl, "V_S' [V]":dbl, "V_L' [V]":dbl, "V_R' [V]":dbl, "V_sum' [V]":dbl, "V_x [V]":dbl, "V_y [V]":dbl, "V_px' [V]":dbl, "V_py' [V]":dbl, "V_pz' [V]":dbl, "dt [s]":dbl, "Vpx_AO [V]":dbl, "Vpy_AO [V]":dbl, "Vpz_AO [V]":dbl, "scan backlog":dbl, "LockInPhase":dbl, "TrapX [nm]":dbl, "TrapY [nm]":dbl, "TrapZ [nm]":dbl, "V_A [V]":dbl, "V_D [V]":dbl, "V_P [V]":dbl, "V_S [V]":dbl, "V_L [V]":dbl, "V_R [V]":dbl, "V_sum [V]":dbl, "V_x [V]":dbl, "V_y [V]":dbl, "P power [mW]":dbl, "S power [mW]":dbl, "angle compensated P power [W]":dbl, "angle compensated S power [W]":dbl, "angle compensated V_L":dbl, "angle compensated V_R":dbl, "angle compensated V_sum [V]":dbl, "angle compensated V_x [V]":dbl, "angle compensated V_y [V]":dbl, "Psi [rad]":dbl, "Laser power before objective[W]":dbl, "E_in":dbl, "E_out":dbl, "Delta E":dbl, "X signal":dbl, "Y signal":dbl, "Z signal":dbl, "TrapX (AO) [nm]":dbl, "TrapY (AO) [nm]":dbl, "TrapZ (AO) [nm]":dbl, "Fz [pN]":dbl, "Zext [nm]":dbl, "Tau [pNnm]":dbl, "Turn":dbl, "Fx [pN]":dbl, "Xext [nm]":dbl, "Fy [pN]":dbl, "Yext [nm]":dbl, "time [s]":dbl, "Delta Z signal":dbl, "Delta Z bead [nm]":dbl, "Z bead [nm]":dbl, "Delta TrapZ [nm]":dbl, "Delta Xsignal":dbl, "X bead [nm]":dbl, "Delta Ysignal":dbl, "Y bead [nm]":dbl, "Stop Condition":dbl}
  T25 = cluster{"folder name":string, "file name":string, "Processed data":T24[]}
  T26 = enum16{"open", "replace", "create", "open or create", "replace or create", "replace or create with confirmation"}
  T27 = cluster{cluster{"trace (folder) name":string, "task (file) name":string, "processed data":T24[]}[], "tasklist (name)":string[], "trace name":string, "description":string, "Array of Params":T3[]}
  T28 = cluster{"trace#":i32, cluster{"index":i32, "File path":path, "File name":string}[], "description":string, "Convert?":bool, "params array":T3[], "Array":refnum<class "Task.lvclass">[]}
  T29 = cluster{cluster{"trace (folder) name":string, "task (file) name":string, "processed data":T24[]}[], "tasklist (name)":string[], "trace name":string, "description":string, "Array of Params":T3[]}[]
  T30 = cluster{"index":i32, "File path":path, "File name":string}[]
  T31 = typedef "SignalConverson.lvlib/Physical Quantitites.ctl" = cluster{"Fz [pN]":dbl, "Zext [nm]":dbl, "Tau [pNnm]":dbl, "Turn":dbl, "Fx [pN]":dbl, "Xext [nm]":dbl, "Fy [pN]":dbl, "Yext [nm]":dbl, "time [s]":dbl, "Delta Z signal":dbl, "Delta Z bead [nm]":dbl, "Z bead [nm]":dbl, "Delta TrapZ [nm]":dbl, "Delta Xsignal":dbl, "X bead [nm]":dbl, "Delta Ysignal":dbl, "Y bead [nm]":dbl, "Stop Condition":dbl}
  T32 = cluster{"index cross = max-1":bool, "index cross = max-2":bool, "index cross = 0":bool, "index cross = 1":bool, "Exceeds max iter":bool, "no solution 2rd order polyn ":bool}
  T33 = cluster{"trace (folder) name":string, "task (file) name":string, "processed data":T24[]}[]
  T34 = cluster{"p":dbl, "l0":dbl, "k0":dbl, "residue":dbl}
  T35 = typedef "Initialization.lvlib/FileManagement.lvlib/Folder information.ctl" = cluster{"Folder index":i32, "Date modefied":i32, "Folder name":string, "Description":string, "Key words":string, "Log in Finding index":string}[]
  T36 = cluster{"Folder index":i32, "dup file":path, string}
  T37 = cluster{"Folder index":i32, "appended path":path, string}
  T38 = cluster{"Folder index":i32, "appended path":path, string}[]
  T39 = cluster{"trace (folder) name":string, "task (file) name":string, "processed data":T24[]}
  T40 = cluster{"X Values":dbl[], "Histogram: h(x)":i32[]}
  T41 = cluster{"X Values":dbl[], "Best Gaussian Fit":dbl[]}
  T42 = typedef "LVPointDoubleTypeDef.ctl" = cluster{"Cursor X":dbl, "Cursor Y":dbl}
  T43 = cluster{string, string, "Flattened data 1D array":T24[]}
  T44 = cluster{cluster{string, string, "Flattened data 1D array":T24[]}[], string[], string, string, "Array of Params const":T3[]}
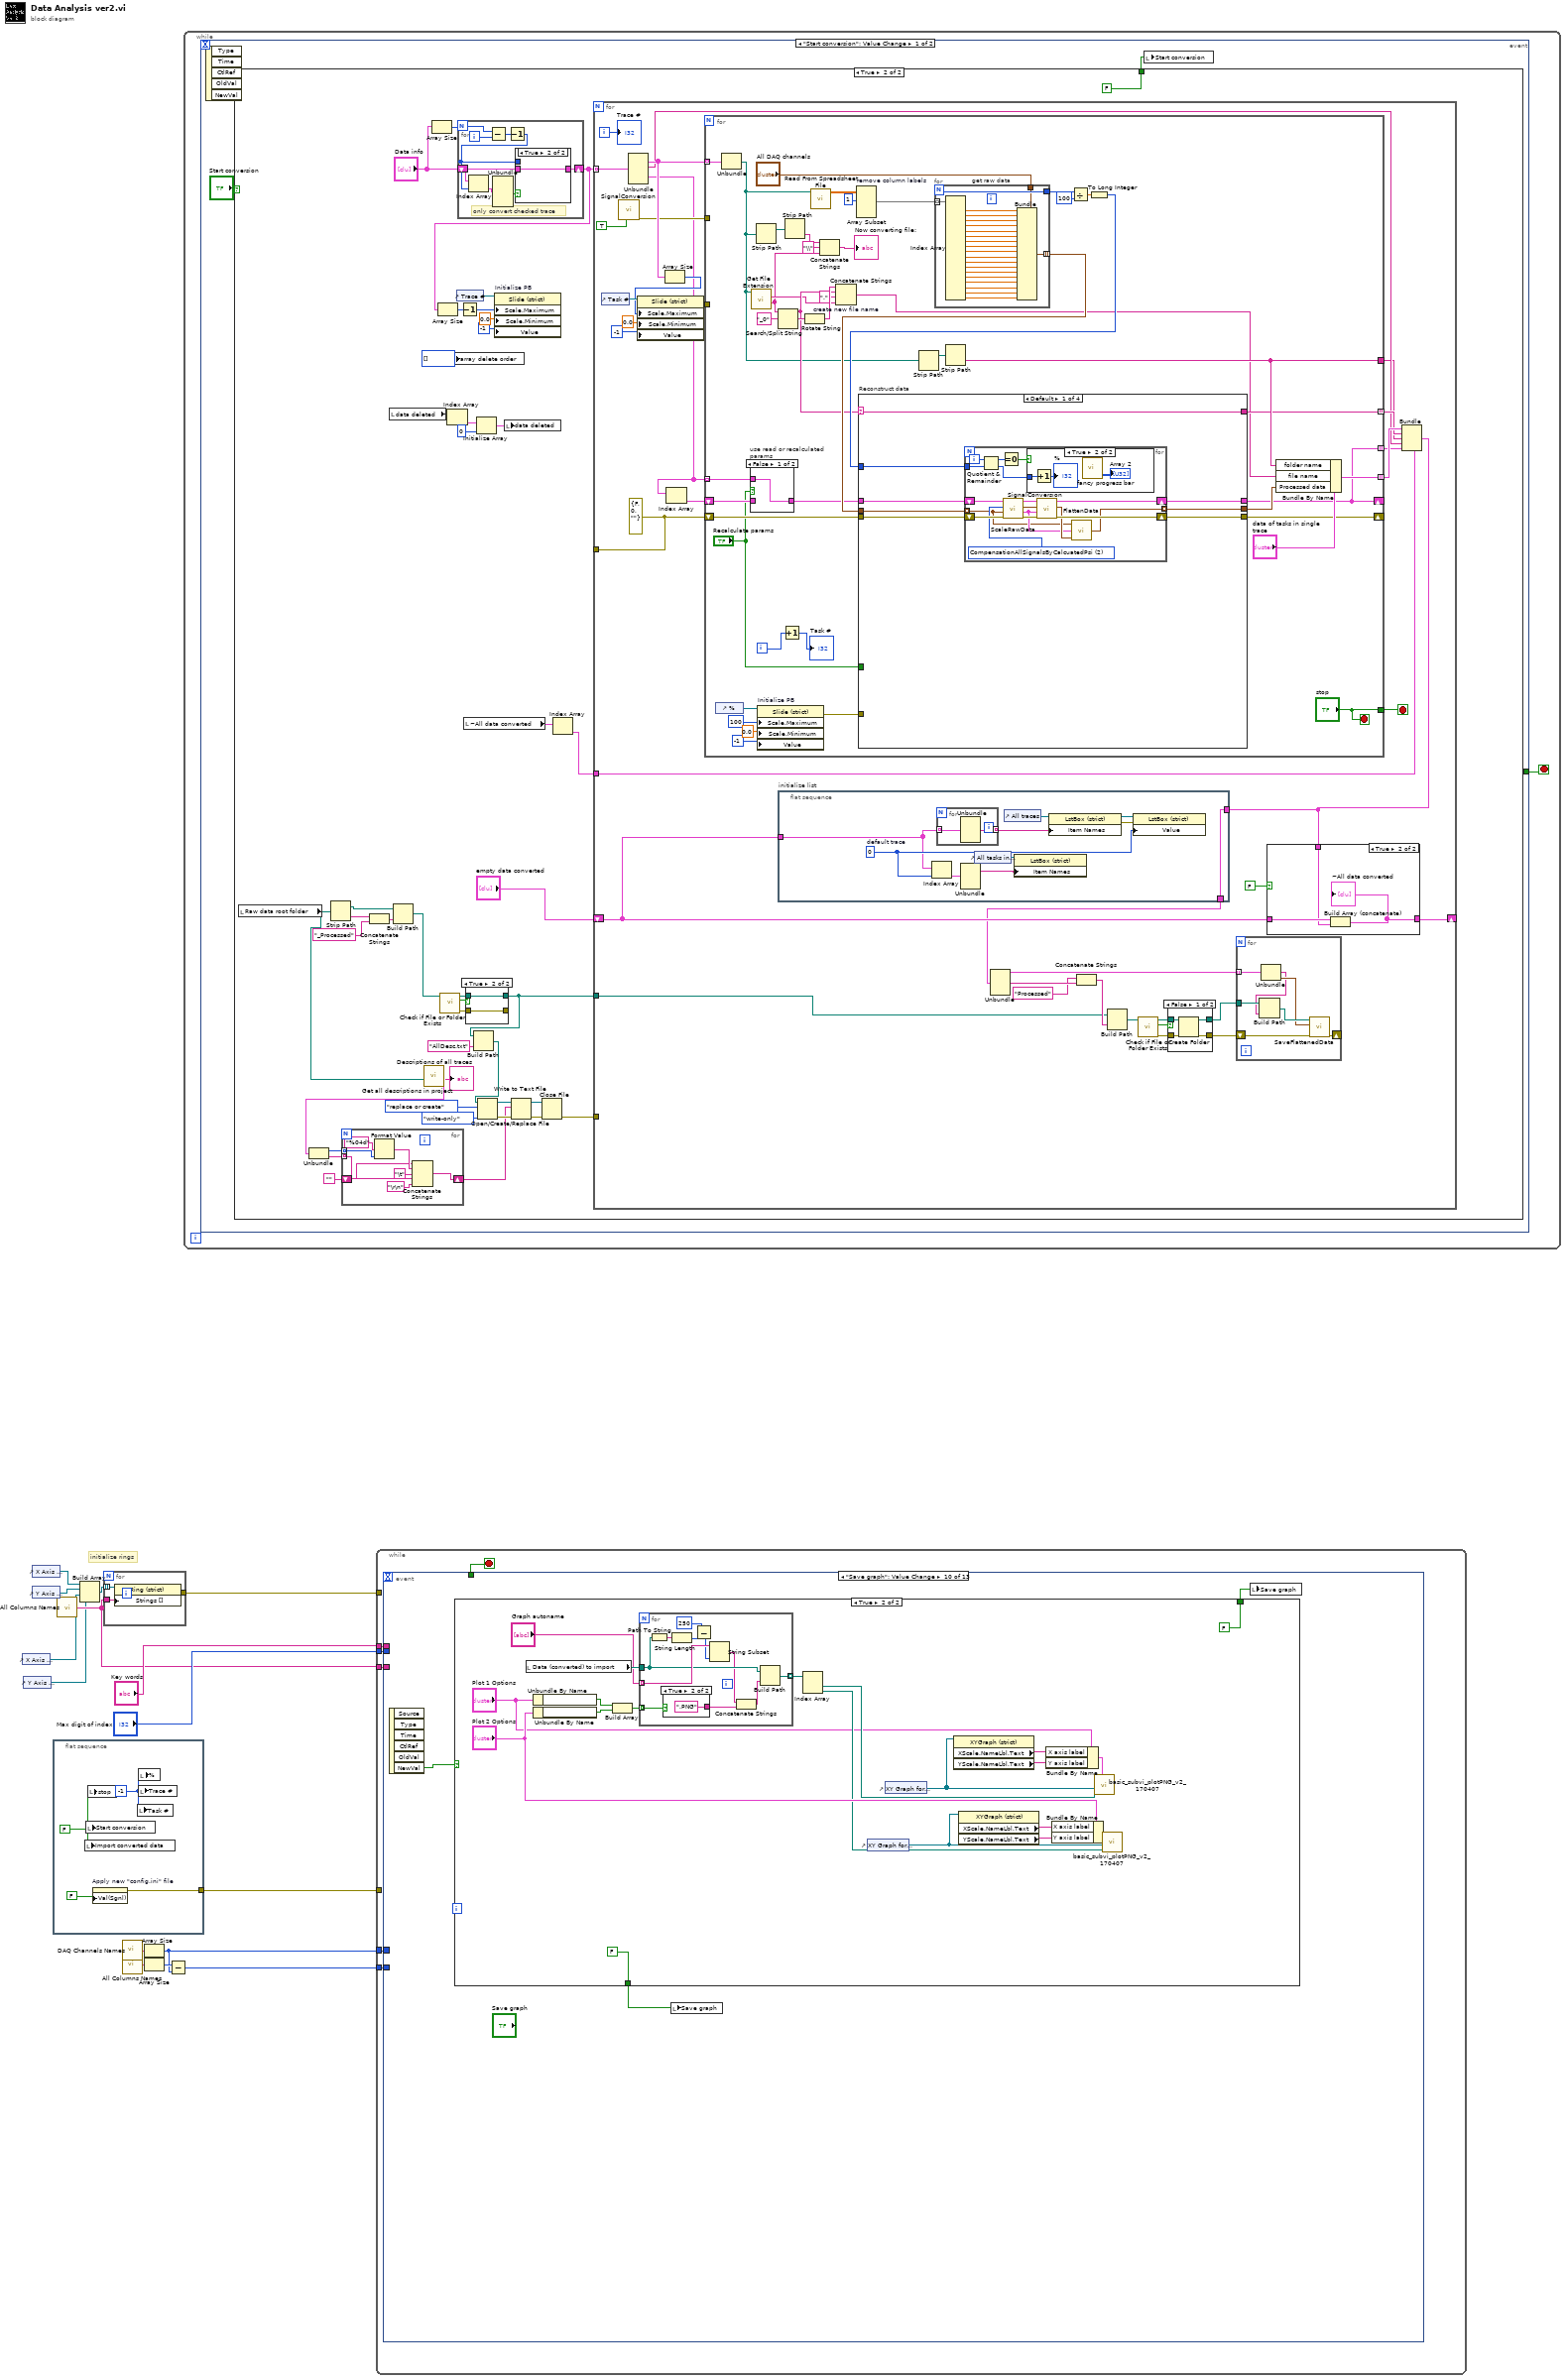
[diagram p0: block diagram]
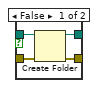
[diagram p3: hidden frame]
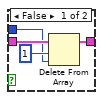
[diagram p4: hidden frame]
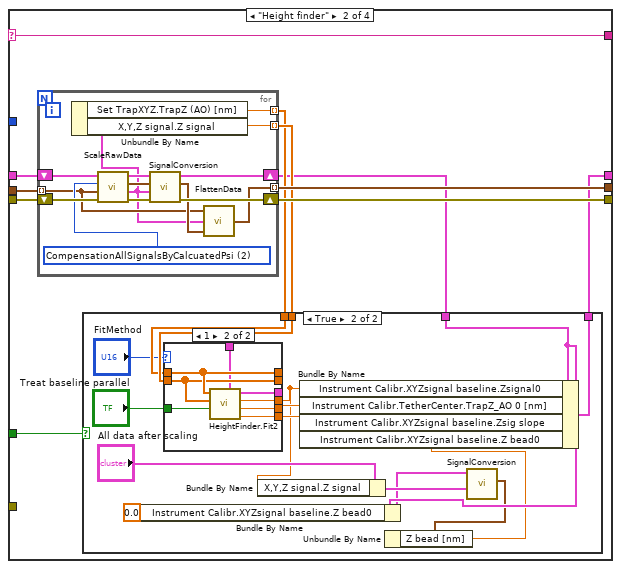
[diagram p9: hidden frame]
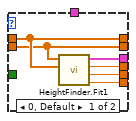
[diagram p11: hidden frame]
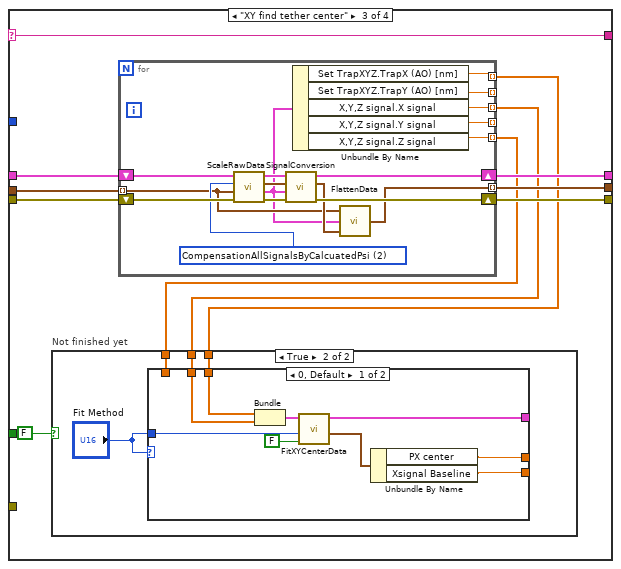
[diagram p12: hidden frame]
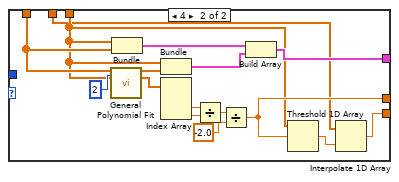
[diagram p14: hidden frame]
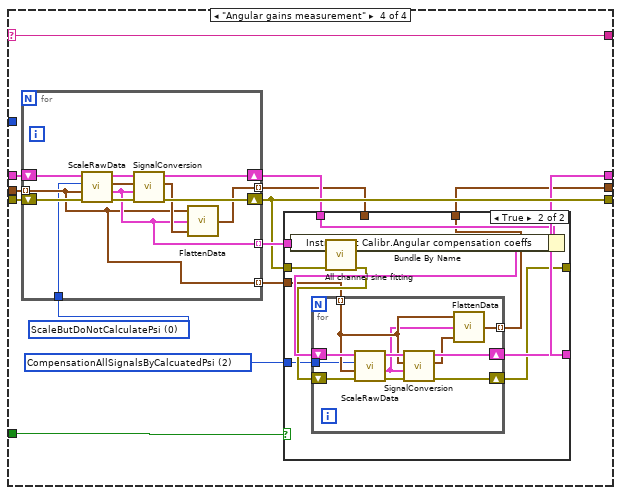
[diagram p15: hidden frame]
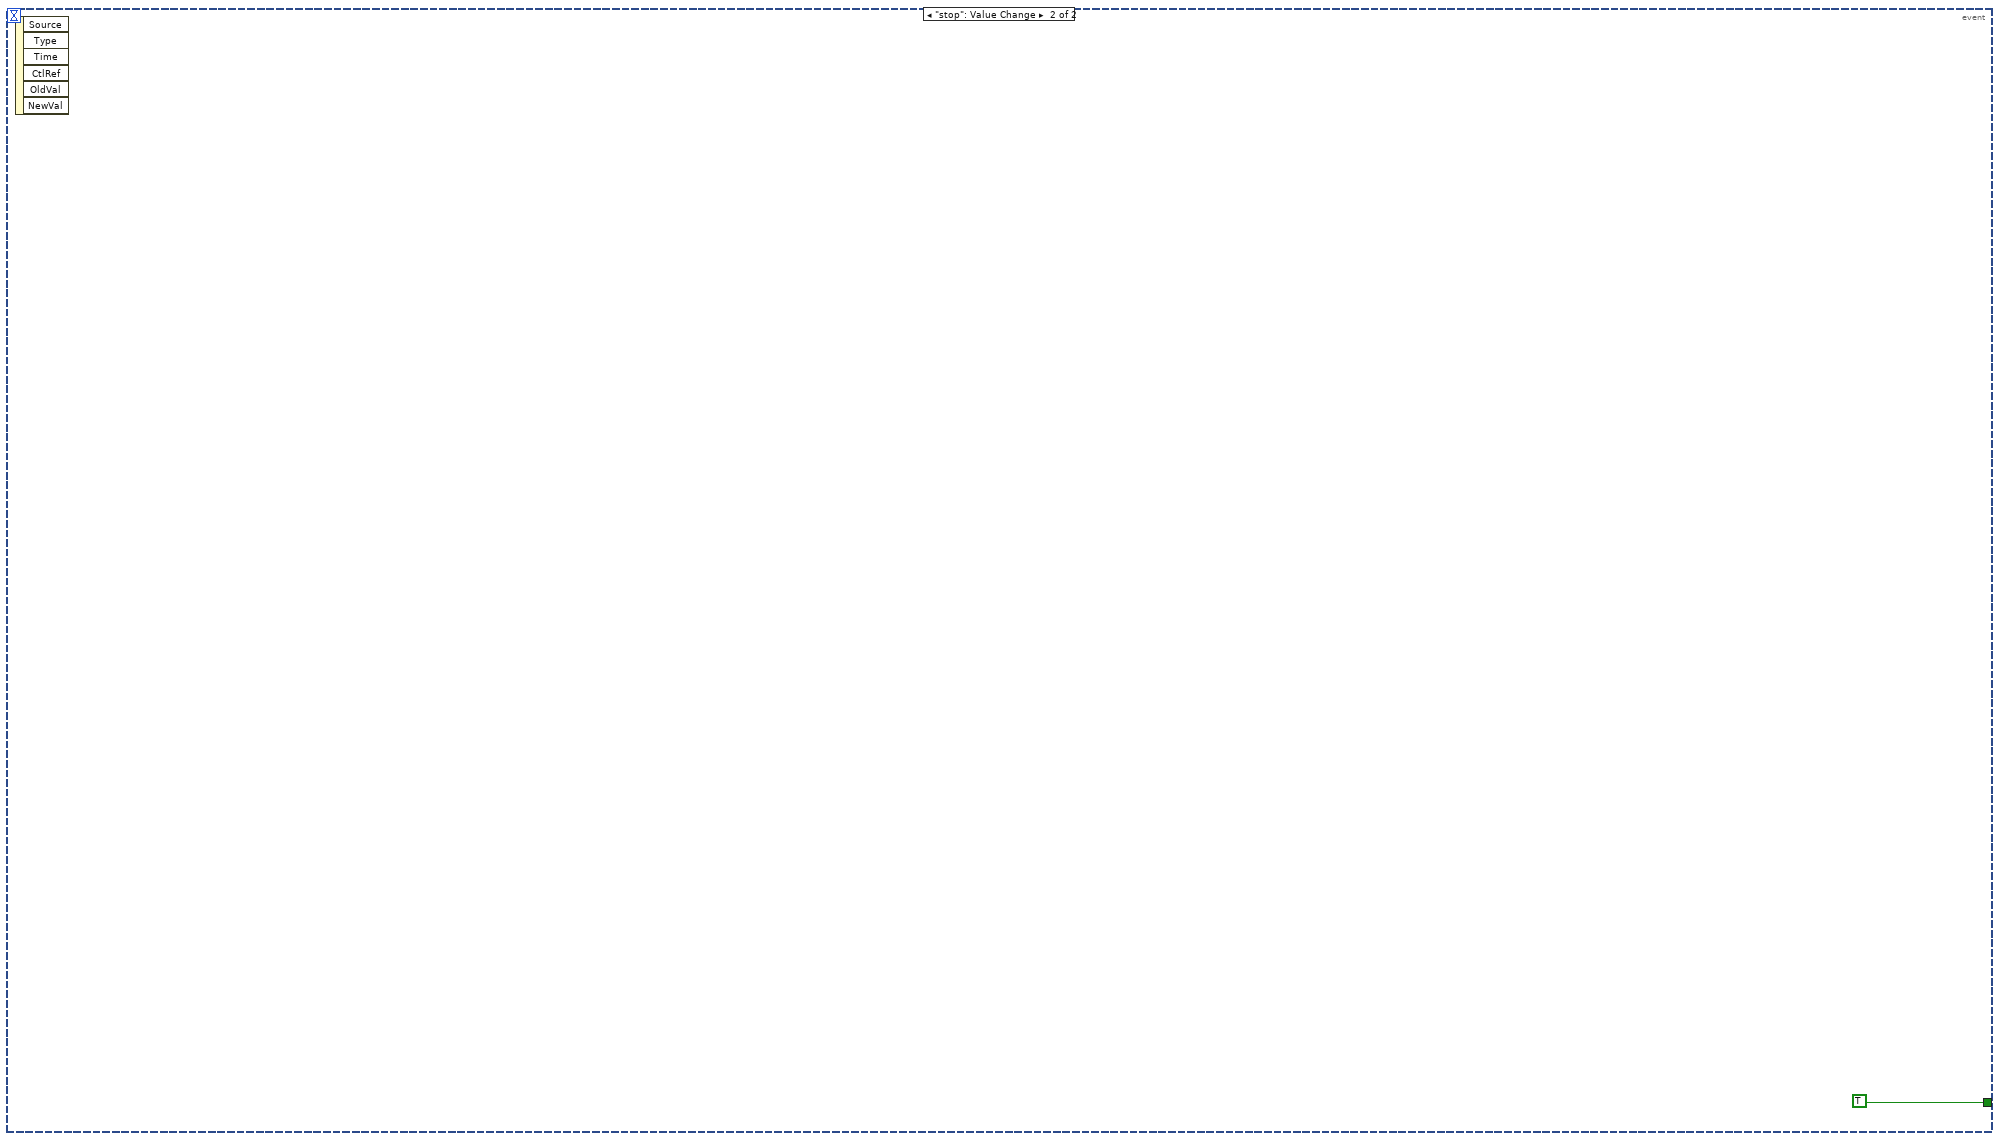
[diagram p17: hidden frame]
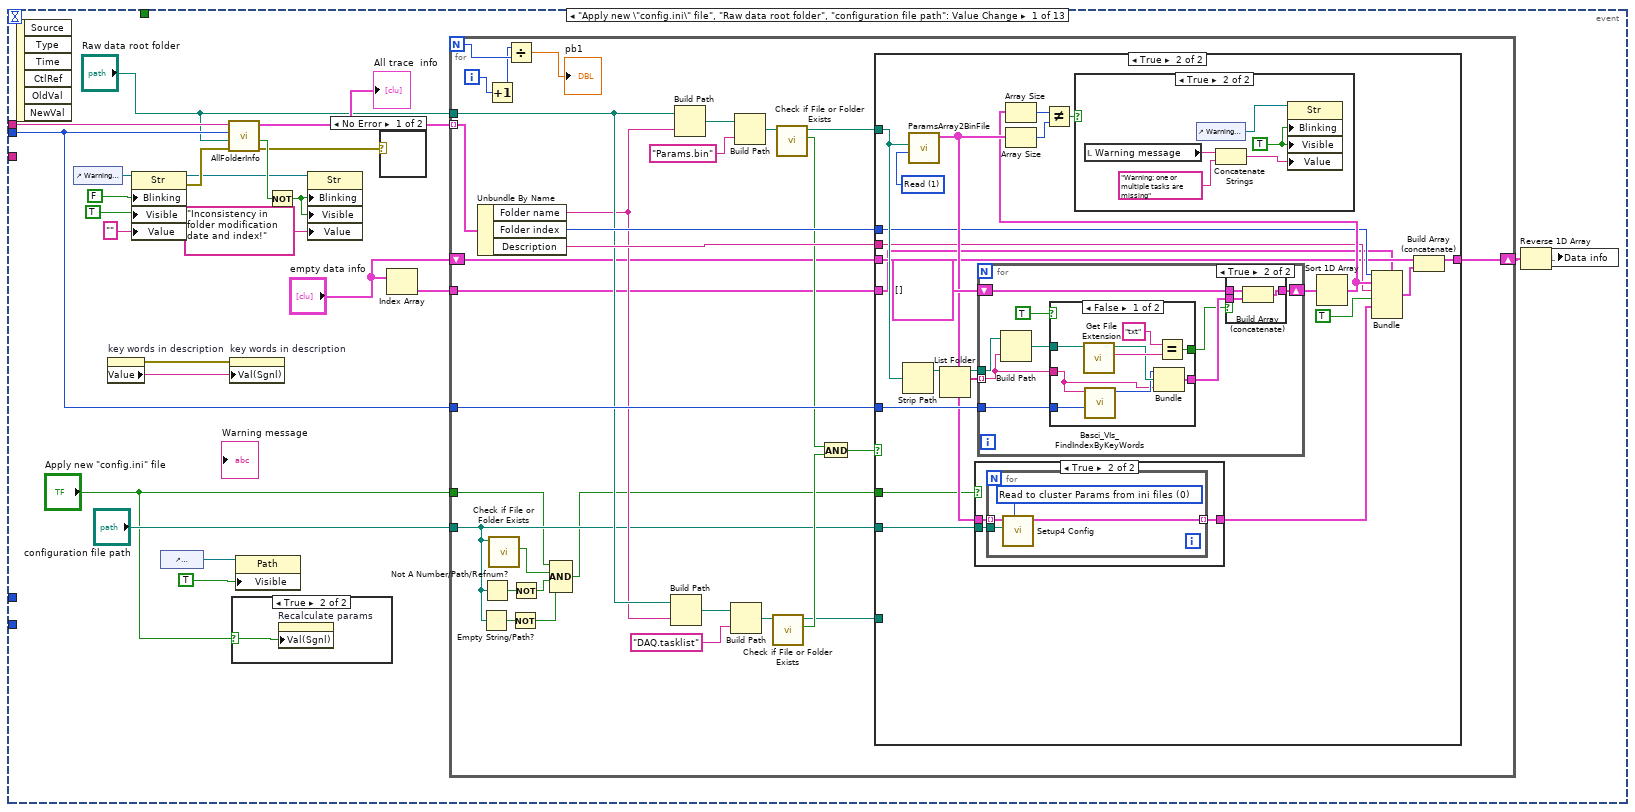
[diagram p18: hidden frame]
diagram:
  # "initialize rings"
  n1 = control-ref of="X Axis to plot 2"() -> (w2:refnum<vi>)
  n2 = control-ref of="Y Axis to plot 2"() -> (w1:refnum<vi>)
  n3 = control-ref of="X Axis to plot"() -> (w6:refnum<vi>)
  n4 = control-ref of="Y Axis to plot"() -> (w7:refnum<vi>)
  n5 = flat-sequence {
    tunnel: [w18] -> w15
    frame #0 {
      w19 = -1 ("%")
      w17 = FALSE ("Start conversion")
      n6 = local write "Import converted data"(w17) -> ()
      n7 = local write "Start conversion"(w17) -> ()
      n8 = local write "stop"(w17) -> ()
      n9 = property on="Apply new \"config.ini\" file" class="Bool (strict)"("Val(Sgnl)"=FALSE ("Blinking")) -> (error out=w18:errorcluster)  [unwired: 2 in, 1 out]
      n10 = local write "Task #"(w19) -> ()
      n11 = local write "Trace #"(w19) -> ()
      n12 = local write "%"(w19) -> ()
    }
  }
  n13 = call "All Columns Names.vi"() -> ("All column names"=w3:string[])
  n14 = Build Array(w6, w7, w2, w1) -> (w5:refnum<vi>[])
  n15 = for {
    tunnel: w5 -> [w22] mode=indexing
    tunnel: w3 -> [w21]
    tunnel: [w20] -> w4
    n16 = property class="Ring (strict)"(reference=w22, "Strings []"=w21) -> (error out=w20:errorcluster)  [unwired: 1 in, 1 out]
  }
  n17 = call "DAQ Channels Names.vi"() -> ("DAQ channel names (string)"=w12:string[])  [unwired: 7 in]
  n18 = call "All Columns Names.vi"() -> ("All column names"=w11:string[])
  n19 = Array Size(array=w12) -> (size(s)=w9:i32)
  n20 = Array Size(array=w11) -> (size(s)=w10:i32)
  n21 = Subtract(x=w10, y=w9) -> (x-y=w8:i32)
  n22 = while {
    stop <- w23 stop-if-true
    n23 = event shown="[0] \"Start conversion\": Value Change" {
      selector: _ -> [_ _]
      dyn-events: _ -> [_ _]
      timeout: _ -> [_ _]
      tunnel: [_ TRUE] -> w23
      event "Start conversion": Value Change {
        n24 = event-data() -> ()  [unwired: 1 in, 5 out]
        n25 = case shown="True" "Start conversion" {
          tunnel: [_ FALSE ("start conversion 2")] -> w25
          frame False {
          }
          frame True {
            n26 = local read "Raw data root folder"() -> (w42:path)
            n27 = Strip Path(path=w42) -> (stripped path=w46:path, name=w48:string)
            n28 = Concatenate Strings(w48, "_Processed" ("string")) -> (w49:string)
            n29 = local read "data deleted"() -> (w57:T23)
            n30 = Build Path(base path=w46, name or relative path=w49) -> (appended path=w50:path)
            n31 = call "Get all descriptions in project.vi"("Folder Path"=w42) -> ("All descriptions"=→"Descriptions of all traces":string, "Descriptions and trace index"=w35:cluster{i32[], string[]})  [unwired: 7 in]
            n32 = Unbundle(w35) -> (w34:i32[], w33:string[])
            n33 = for {
              tunnel: w34 -> [w75] mode=indexing
              tunnel: w33 -> [w72] mode=indexing
              shift-right: [w69] -> w31
              shift-left: "" -> [w68]
              n34 = Format Value(format string="%04d" ("string (\"\")"), value (0)=w75) -> (output string=w73:string)  [unwired: 1 in]
              n35 = Concatenate Strings(w68, w73, "\t", w72, "\r\n") -> (w69:string)
            }
            n36 = Array Size(array="Data info") -> (size(s)=w65:i32)
            n37 = call <vilib>:"Check if File or Folder Exists.vi"("path"=w50) -> ("error out"=w45:errorcluster, "file or folder exists?"=w43:bool, "dup path"=w44:path)  [unwired: 8 in]
            n38 = Index Array(array=w57) -> (element=w56:T27)  [unwired: 1 in]
            n39 = local write "array delete order"(i32[] [] ("array delete order")) -> ()
            n40 = control-ref of="Trace #"() -> (w63:refnum<vi>)
            n41 = for {
              N: w65 -> [w88]
              shift-right: [w89] -> w59
              shift-left: "Data info" -> [w85]
              i -> [w87]
              # "only convert checked trace"
              n42 = Subtract(x=w88, y=w87) -> (x-y=w86:i32)
              n43 = Decrement(x=w86) -> (x-1=w82:i32)
              n44 = Index Array(array=w85, index=w82) -> (element=w84:T28)
              n45 = Unbundle(w84) -> ("Convert?"=w83:bool)  [unwired: 5 out]
              n46 = case shown="True" w83 {
                tunnel: w85 -> [w93 w94]
                tunnel: [w92 w94] -> w89
                tunnel: w82 -> [w90 _]
                frame False {
                  n47 = Delete From Array(array=w93, length=1, index=w90) -> (array with subset deleted=w92:T2)  [unwired: 1 out]
                }
                frame True {
                }
              }
            }
            n48 = Array Size(array=w59) -> (size(s)=w64:i32)
            n49 = Decrement(x=w64) -> (x-1=w60:i32)
            n50 = local read "~All data converted"() -> (w53:T23)
            n51 = case shown="True" w43 {
              tunnel: [w79 w81] -> w41
              tunnel: [w78 w80] -> _
              tunnel: w45 -> [w77 w80]
              tunnel: w44 -> [w76 w81]
              frame False {
                n52 = Create Folder(path (use dialog)=w76, error in=w77) -> (created path=w79:path, error out=w78:errorcluster)  [unwired: 1 in, 1 out]
              }
              frame True {
              }
            }
            n53 = Build Path(base path=w41, name or relative path="AllDesc.txt") -> (appended path=w39:path)
            n54 = Initialize Array(w56, 0 ("dimension size")) -> (w54:T29)
            n55 = Open/Create/Replace File(file path (use dialog)=w39, operation (0:open)=T26."replace or create", access (0:read/write)=enum16{"read/write", "read-only", "write-only"}."write-only") -> (refnum out=w29:refnum<file>, error out=w36:errorcluster)  [unwired: 3 in, 1 out]
            n56 = property on="Initialize PB" class="Slide (strict)"(reference=w63, "Scale.Maximum"=w60, "Scale.Minimum"=0.0 ("Scale.Range:Minimum"), "Value"=-1 ("标尺.范围:最小值")) -> ()  [unwired: 1 in, 2 out]
            n57 = local write "data deleted"(w54) -> ()
            n58 = Write to Text File(file (use dialog)=w29, text=w31, error in=w36) -> (refnum out=w27:refnum<file>, error out=w28:errorcluster)  [unwired: 1 in, 1 out]
            n59 = Close File(refnum=w27, error in=w28) -> (error out=w26:errorcluster)  [unwired: 1 out]
            n60 = Index Array(array=w53) -> (element=w52:T27)  [unwired: 1 in]
            n61 = for {
              tunnel: w59 -> [w124] mode=indexing
              tunnel: w52 -> [w112]
              shift-right: [w111] -> _
              shift-left: "empty data converted" -> [w110]
              tunnel: [w109] -> _
              tunnel: w41 -> [w98]
              tunnel: w26 -> [_]
              i -> [w127]
              stop <- w125 stop-if-true
              w109 = errorcluster {"status"=FALSE, "code"=0, "source"=""} ("error out")
              n62 = control-ref of="Task #"() -> (w130:refnum<vi>)
              n63 = call "SignalConversion.vi"("Reinitialize time? (F)"=TRUE) -> ("error out"=w121:errorcluster)  [unwired: 6 in, 4 out]
              n64 = Unbundle(w124) -> (w122:T30, "description"=w117:string, "params array"=w116:T3[])  [unwired: 3 out]
              n65 = Array Size(array=w122) -> (size(s)=w123:i32)
              n66 = property on="属性节点" class="Slide (strict)"(reference=w130, "Scale.Maximum"=w123, "Scale.Minimum"=0.0 ("Scale.Range:Minimum"), "Value"=-1 ("标尺.范围:最小值")) -> (error out=w126:errorcluster)  [unwired: 1 in, 1 out]
              n67 = Index Array(array=w116) -> (element=w115:T3)  [unwired: 1 in]
              n68 = for {
                tunnel: w122 -> [w197] mode=indexing
                tunnel: [w196] -> w113
                tunnel: [w182] -> w118 mode=indexing
                tunnel: w126 -> [_]
                tunnel: ["stop"] -> w125
                tunnel: w116 -> [w180] mode=indexing
                tunnel: w121 -> [_]
                tunnel: [w193] -> w119 mode=indexing
                shift-right: [w177] -> _
                shift-left: w115 -> [w179]
                shift-right: [w184] -> _
                shift-left: w109 -> [w185]
                tunnel: [w177] -> w114 mode=indexing
                i -> [w167]
                stop <- "stop" stop-if-true
                n69 = control-ref of="%"() -> (w201:refnum<vi>)
                n70 = Unbundle(w197) -> ("File path"=w165:path)  [unwired: 2 out]
                n71 = case "use read or recalculated params" shown="False" "Recalculate params" {
                  tunnel: w180 -> [w204 _]
                  tunnel: [w204 w205] -> w178
                  tunnel: w179 -> [_ w205]
                  frame False {
                  }
                  frame True {
                  }
                }
                n72 = call <vilib>:"Get File Extension.vi"("file"=w165) -> ("filename without extension"=w163:string, "lowercase file extension"=w170:string)  [unwired: 6 in, 3 out]
                n73 = Strip Path(path=w165) -> (stripped path=w164:path)  [unwired: 1 out]
                n74 = property on="Initialize PB" class="Slide (strict)"(reference=w201, "Scale.Maximum"=100 ("y"), "Scale.Minimum"=0.0 ("Scale.Range:Minimum"), "Value"=-1 ("标尺.范围:最小值")) -> (error out=w181:errorcluster)  [unwired: 1 in, 1 out]
                n75 = Search/Split String(string=w163, search string/char (-)="_0") -> (substring before match=w171:string, match + rest of string=w173:string)  [unwired: 1 in, 1 out]
                n76 = Increment(x=w167) -> (x+1=→"Task #":i32)
                n77 = Strip Path(path=w164) -> (name=w161:string)  [unwired: 1 out]
                n78 = Rotate String(1:w173) -> (0:w172:string)
                n79 = call-poly <vilib>:"Read From Spreadsheet File.vi"("file path (dialog if empty)"=w165) -> ("all rows"=w194:dbl[][])  [unwired: 6 in, 4 out]
                n80 = Concatenate Strings(w161, "\\" ("string"), w163) -> (→"Now converting file:":string)
                n81 = Concatenate Strings "create new file name"(w172, w171, "." ("string"), w170) -> (w169:string)
                n82 = Array Subset "remove column labels"(array=w194, index (row)=1 ("index")) -> (w191:dbl[][])  [unwired: 3 in]
                n83 = Strip Path(path=w165) -> (stripped path=w202:path)  [unwired: 1 out]
                n84 = for "get raw data" {
                  N -> [w398]
                  tunnel: w191 -> [w401] mode=indexing
                  tunnel: [w399] -> w186 mode=indexing
                  tunnel: [w398] -> w189
                  tunnel: "All DAQ channels" -> [w397]
                  n85 = Index Array(array=w401) -> (element #1=w402:dbl, element #2=w403:dbl, element #3=w404:dbl, element #4=w405:dbl, element #5=w406:dbl, element #6=w407:dbl, element #7=w408:dbl, element #8=w409:dbl, element #9=w410:dbl, element #10=w411:dbl, element #11=w412:dbl, element #12=w413:dbl, element #13=w414:dbl, element #14=w415:dbl, element #15=w416:dbl, element #16=w417:dbl, element #17=w418:dbl, element #18=w400:dbl)  [unwired: 18 in]
                  n86 = Bundle(cluster=w397, "V_A' [V]"=w402, "V_D' [V]"=w403, "V_P'  [V]"=w404, "V_S' [V]"=w405, "V_L' [V]"=w406, "V_R' [V]"=w407, "V_sum' [V]"=w408, "V_x [V]"=w409, "V_y [V]"=w410, "V_px' [V]"=w411, "V_py' [V]"=w412, "V_pz' [V]"=w413, "dt [s]"=w414, "Vpx_AO [V]"=w415, "Vpy_AO [V]"=w416, "Vpz_AO [V]"=w417, "scan backlog"=w418, "LockInPhase"=w400) -> (w399:T22)
                }
                n87 = Strip Path(path=w202) -> (name=w196:string)  [unwired: 1 out]
                n88 = Divide(x=w189, y=100) -> (x/y=w190:dbl)
                n89 = To Long Integer(number=w190) -> (32bit integer=w187:i32)
                n90 = case "Reconstruct data" shown="Default" w171 {
                  selector: w171 -> [w206 w239 w293 w356]
                  tunnel: w187 -> [w213 _ _ _]
                  tunnel: w186 -> [w212 w244 w299 w359]
                  tunnel: [w211 w234 w298 w350] -> w177
                  tunnel: [w210 w243 w297 w353] -> w184
                  tunnel: w185 -> [w209 w242 w296 w358]
                  tunnel: w178 -> [w208 w241 w295 w357]
                  tunnel: [w207 w240 w294 w348] -> w183
                  tunnel: [w206 w239 w293 w356] -> w182
                  tunnel: w181 -> [_ _ _ _]
                  tunnel: "Recalculate params" -> [_ w236 _ w354]
                  frame Default {
                    n91 = for {
                      shift-right: [w226] -> w210
                      shift-left: w209 -> [w227]
                      shift-right: [w225] -> w211
                      shift-left: w208 -> [w230]
                      tunnel: w213 -> [w224]
                      tunnel: [w218] -> w207 mode=indexing
                      tunnel: w212 -> [w214] mode=indexing
                      i -> [w223]
                      w215 = 2 items=["ScaleButDoNotCalculatePsi", "CalculatePsi, ButDoNotCompensate", "CompensationAllSignalsByCalcuatedPsi", "DoNotScale(ReadRawVoltageSignals)"] ("Scale Option")
                      n92 = Quotient & Remainder(x=w223, y=w224) -> (x-y*floor(x/y)=w222:i32, floor(x/y)=w220:i32)
                      n93 = Equal To 0?(x=w222) -> (x = 0?=w221:bool)
                      n94 = call "ScaleRawData.vi"("error in (no error)"=w227, "All DAQ channels"=w214, "Scale Option"=w215, "Params in"=w230) -> ("error out"=w228:errorcluster, "Scaled data"=w216:T16, "All DAQ channels out"=w219:T22, "Params out"=w229:T3)  [unwired: 1 in]
                      n95 = case shown="True" w221 {
                        tunnel: w220 -> [_ w233]
                        frame False {
                        }
                        frame True {
                          n96 = Increment(x=w233) -> (x+1=→"%":i32)
                          n97 = call "fancy progress bar.vi"() -> ("Array 2"=→"Array 2":u32[][])  [unwired: 1 in, 1 out]
                        }
                      }
                      n98 = call "SignalConversion.vi"("error in (no error)"=w228, "All data after scaling"=w216, "All DAQ channels"=w219, "Params in"=w229) -> ("error out"=w226:errorcluster, "Physical Quantities cluster out"=w217:T31, "Params out"=w225:T3)  [unwired: 3 in, 2 out]
                      n99 = call "FlattenData.vi"("Physical Quantities"=w217, "All data after scaling"=w216, "All DAQ channels"=w214) -> ("Flattened data"=w218:T24)  [unwired: 2 in]
                    }
                  }
                  frame "Height finder" {
                    n100 = for {
                      shift-right: [w284] -> w243
                      shift-left: w242 -> [w285]
                      shift-right: [w283] -> w235
                      shift-left: w241 -> [w288]
                      tunnel: [w281] -> w240 mode=indexing
                      tunnel: w244 -> [w278] mode=indexing
                      tunnel: [w276] -> w238 mode=indexing
                      tunnel: [w275] -> w237 mode=indexing
                      w279 = 2 items=["ScaleButDoNotCalculatePsi", "CalculatePsi, ButDoNotCompensate", "CompensationAllSignalsByCalcuatedPsi", "DoNotScale(ReadRawVoltageSignals)"] ("Scale Option")
                      n101 = call "ScaleRawData.vi"("error in (no error)"=w285, "All DAQ channels"=w278, "Scale Option"=w279, "Params in"=w288) -> ("error out"=w286:errorcluster, "Scaled data"=w277:T16, "All DAQ channels out"=w282:T22, "Params out"=w287:T3)  [unwired: 1 in]
                      n102 = Unbundle By Name(w277) -> ("Set TrapXYZ.TrapZ (AO) [nm]"=w275:dbl, "X,Y,Z signal.Z signal"=w276:dbl)
                      n103 = call "SignalConversion.vi"("error in (no error)"=w286, "All data after scaling"=w277, "All DAQ channels"=w282, "Params in"=w287) -> ("error out"=w284:errorcluster, "Physical Quantities cluster out"=w280:T31, "Params out"=w283:T3)  [unwired: 3 in, 2 out]
                      n104 = call "FlattenData.vi"("Physical Quantities"=w280, "All data after scaling"=w277, "All DAQ channels"=w278) -> ("Flattened data"=w281:T24)  [unwired: 2 in]
                    }
                    n105 = case shown="True" w236 {
                      tunnel: w238 -> [_ w260]
                      tunnel: w237 -> [_ w259]
                      tunnel: w235 -> [w245 w249]
                      tunnel: [w245 w250] -> w234
                      frame False {
                      }
                      frame True {
                        n106 = Bundle By Name(cluster=w249, "Instrument Calibr.XYZsignal baseline.Z bead0"=0.0) -> (w248:T3)
                        n107 = case shown="1" "FitMethod" {
                          tunnel: w259 -> [w265 w272]
                          tunnel: w260 -> [w264 w271]
                          tunnel: [w266 w274] -> _
                          tunnel: [w263 w273] -> w256
                          tunnel: [w265 w272] -> _
                          tunnel: [w264 w271] -> _
                          tunnel: [w262 w270] -> w252
                          tunnel: [_ w269] -> _
                          tunnel: [w261 w268] -> w255
                          tunnel: "Treat baseline parallel" -> [_ w267]
                          frame 0, Default {
                            n108 = call "HeightFinder.Fit1.vi"("X"=w265, "Y"=w264) -> ("Zsig slope vs Pz"=w261:dbl, "Bottom Position"=w263:dbl, "Z signal basline"=w262:dbl, "Display result"=w266:cluster{"Y":dbl[], "Y":dbl[]}[])  [unwired: 2 in]
                          }
                          frame 1 {
                            n109 = call "HeightFinder.Fit2.vi"("TrapZ"=w272, "Vsum or Z signal"=w271, "Treat baseline parallel"=w267) -> ("Error in fitting"=w269:T32, "XY plot"=w274:cluster{dbl[], dbl[]}[], "Z signal baseline"=w270:dbl, "bottom position"=w273:dbl, "Z signal slope (vs Pz output)"=w268:dbl)  [unwired: 2 out]
                          }
                        }
                        n110 = Bundle By Name(cluster="All data after scaling", "X,Y,Z signal.Z signal"=w252) -> (w253:T16)
                        n111 = call "SignalConversion.vi"("All data after scaling"=w253, "Params in"=w248) -> ("Physical Quantities cluster out"=w247:T31)  [unwired: 5 in, 4 out]
                        n112 = Unbundle By Name(w247) -> ("Z bead [nm]"=w246:dbl)
                        n113 = Bundle By Name(cluster=w249, "Instrument Calibr.XYZsignal baseline.Zsignal0"=w252, "Instrument Calibr.TetherCenter.TrapZ_AO 0 [nm]"=w256, "Instrument Calibr.XYZsignal baseline.Zsig slope"=w255, "Instrument Calibr.XYZsignal baseline.Z bead0"=w246) -> (w250:T3)
                      }
                    }
                  }
                  frame "XY find tether center" {
                    n114 = for {
                      shift-right: [w341] -> w297
                      shift-left: w296 -> [w342]
                      shift-right: [w340] -> w298
                      shift-left: w295 -> [w345]
                      tunnel: [w338] -> w294 mode=indexing
                      tunnel: w299 -> [w335] mode=indexing
                      tunnel: [w333] -> w291 mode=indexing
                      tunnel: [w332] -> _ mode=indexing
                      tunnel: [w331] -> w290 mode=indexing
                      tunnel: [w330] -> _ mode=indexing
                      tunnel: [w329] -> w292 mode=indexing
                      w336 = 2 items=["ScaleButDoNotCalculatePsi", "CalculatePsi, ButDoNotCompensate", "CompensationAllSignalsByCalcuatedPsi", "DoNotScale(ReadRawVoltageSignals)"] ("Scale Option")
                      n115 = call "ScaleRawData.vi"("error in (no error)"=w342, "All DAQ channels"=w335, "Scale Option"=w336, "Params in"=w345) -> ("error out"=w343:errorcluster, "Scaled data"=w334:T16, "All DAQ channels out"=w339:T22, "Params out"=w344:T3)  [unwired: 1 in]
                      n116 = call "SignalConversion.vi"("error in (no error)"=w343, "All data after scaling"=w334, "All DAQ channels"=w339, "Params in"=w344) -> ("error out"=w341:errorcluster, "Physical Quantities cluster out"=w337:T31, "Params out"=w340:T3)  [unwired: 3 in, 2 out]
                      n117 = Unbundle By Name(w334) -> ("Set TrapXYZ.TrapX (AO) [nm]"=w333:dbl, "Set TrapXYZ.TrapY (AO) [nm]"=w332:dbl, "X,Y,Z signal.X signal"=w331:dbl, "X,Y,Z signal.Y signal"=w330:dbl, "X,Y,Z signal.Z signal"=w329:dbl)
                      n118 = call "FlattenData.vi"("Physical Quantities"=w337, "All data after scaling"=w334, "All DAQ channels"=w335) -> ("Flattened data"=w338:T24)  [unwired: 2 in]
                    }
                    n119 = case "Not finished yet" shown="True" FALSE {
                      tunnel: w292 -> [_ w302]
                      tunnel: w291 -> [_ w301]
                      tunnel: w290 -> [_ w300]
                      frame False {
                      }
                      frame True {
                        n120 = case shown="0, Default" "Fit Method" {
                          tunnel: w301 -> [w312 w316]
                          tunnel: w300 -> [w311 w314]
                          tunnel: "Fit Method" -> [w309 _]
                          tunnel: [w306 w328] -> _
                          tunnel: [w305 w317] -> _
                          tunnel: [w304 w313] -> _
                          tunnel: w302 -> [_ w318]
                          frame 0, Default {
                            n121 = Bundle(w312, w311) -> (w310:cluster{dbl[], dbl[]})  [unwired: 1 in]
                            n122 = call "FitXYCenterData.vi"("True  data <-> Simulation\nOff: True data\nOn: Simulated data"=FALSE ("True  data <-> Simulation\nOff: True data\nOn: Simulated data"), "Fit Method"=w309, "Data input"=w310) -> ("Parameters"=w307:cluster{"PX center":dbl, "Xsignal Baseline":dbl}, "data and fit"=w306:cluster{dbl[], "Best Polynomial Fit":dbl[]}[])  [unwired: 1 in, 2 out]
                            n123 = Unbundle By Name(w307) -> ("PX center"=w305:dbl, "Xsignal Baseline"=w304:dbl)
                          }
                          frame 4 {
                            n124 = call <vilib>:"General Polynomial Fit.vi"("Y"=w318, "polynomial order"=2, "X"=w316) -> ("Best Polynomial Fit"=w326:dbl[], "Polynomial Coefficients"=w323:dbl[])  [unwired: 9 in, 2 out]
                            n125 = Bundle(w316, w318) -> (w327:cluster{dbl[], dbl[]})  [unwired: 1 in]
                            n126 = Bundle(w316, "Best Polynomial Fit"=w326) -> (w325:cluster{dbl[], "Best Polynomial Fit":dbl[]})  [unwired: 1 in]
                            n127 = Index Array(array=w323) -> (element #2=w322:dbl, element #3=w321:dbl)  [unwired: 3 in, 1 out]
                            n128 = Divide(x=w322, y=w321) -> (x/y=w320:dbl)
                            n129 = Divide(x=w320, y=-2.0) -> (x/y=w317:dbl)
                            n130 = Build Array(w327, w325) -> (w328:cluster{dbl[], "Best Polynomial Fit":dbl[]}[])
                            n131 = Threshold 1D Array(2:w317, 3:w316) -> (0:w315:dbl)  [unwired: 1 in]
                            n132 = Interpolate 1D Array(1:w315, 2:w314) -> (0:w313:dbl)
                          }
                        }
                      }
                    }
                  }
                  frame "Angular gains measurement" {
                    w346 = 2 items=["ScaleButDoNotCalculatePsi", "CalculatePsi, ButDoNotCompensate", "CompensationAllSignalsByCalcuatedPsi", "DoNotScale(ReadRawVoltageSignals)"] ("Scale Option")
                    w347 = 0 items=["ScaleButDoNotCalculatePsi", "CalculatePsi, ButDoNotCompensate", "CompensationAllSignalsByCalcuatedPsi", "DoNotScale(ReadRawVoltageSignals)"] ("Scale Option")
                    n133 = for {
                      shift-right: [w392] -> w353
                      shift-left: w358 -> [w393]
                      shift-right: [w391] -> w351
                      shift-left: w357 -> [w396]
                      tunnel: [w389] -> w349 mode=indexing
                      tunnel: w359 -> [w386] mode=indexing
                      tunnel: [w387] -> w355 mode=indexing
                      tunnel: [w386] -> w352 mode=indexing
                      tunnel: w347 -> [w385]
                      n134 = call "ScaleRawData.vi"("error in (no error)"=w393, "All DAQ channels"=w386, "Scale Option"=w385, "Params in"=w396) -> ("error out"=w394:errorcluster, "Scaled data"=w387:T16, "All DAQ channels out"=w390:T22, "Params out"=w395:T3)  [unwired: 1 in]
                      n135 = call "SignalConversion.vi"("error in (no error)"=w394, "All data after scaling"=w387, "All DAQ channels"=w390, "Params in"=w395) -> ("error out"=w392:errorcluster, "Physical Quantities cluster out"=w388:T31, "Params out"=w391:T3)  [unwired: 3 in, 2 out]
                      n136 = call "FlattenData.vi"("Physical Quantities"=w388, "All data after scaling"=w387, "All DAQ channels"=w386) -> ("Flattened data"=w389:T24)  [unwired: 2 in]
                    }
                    n137 = case shown="True" w354 {
                      tunnel: w355 -> [_ w373]
                      tunnel: w353 -> [w362 w372]
                      tunnel: [w362 w366] -> _
                      tunnel: w351 -> [w361 w371]
                      tunnel: w352 -> [_ w365]
                      tunnel: [w361 w368] -> w350
                      tunnel: w349 -> [w360 _]
                      tunnel: [w360 w363] -> w348
                      tunnel: w346 -> [_ w364]
                      frame False {
                      }
                      frame True {
                        n138 = call "All channel sine fitting.vi"("error in"=w372, "scaled data array"=w373) -> ("error out"=w367:errorcluster, "best fit parameters"=w370:dbl[][])  [unwired: 2 in, 2 out]
                        n139 = Bundle By Name(cluster=w371, "Instrument Calibr.Angular compensation coeffs"=w370) -> (w369:T3)
                        n140 = for {
                          shift-right: [w381] -> w368
                          shift-left: w369 -> [w384]
                          shift-right: [w380] -> w366
                          shift-left: w367 -> [w383]
                          tunnel: w365 -> [w378] mode=indexing
                          tunnel: w364 -> [w375]
                          tunnel: [w374] -> w363 mode=indexing
                          n141 = call "ScaleRawData.vi"("error in (no error)"=w383, "All DAQ channels"=w378, "Scale Option"=w375, "Params in"=w384) -> ("error out"=w379:errorcluster, "Scaled data"=w376:T16, "Params out"=w382:T3)  [unwired: 1 in, 1 out]
                          n142 = call "SignalConversion.vi"("error in (no error)"=w379, "All data after scaling"=w376, "All DAQ channels"=w378, "Params in"=w382) -> ("error out"=w380:errorcluster, "Physical Quantities cluster out"=w377:T31, "Params out"=w381:T3)  [unwired: 3 in, 2 out]
                          n143 = call "FlattenData.vi"("Physical Quantities"=w377, "All data after scaling"=w376, "All DAQ channels"=w378) -> ("Flattened data"=w374:T24)  [unwired: 2 in]
                        }
                      }
                    }
                  }
                }
                n144 = Bundle By Name(cluster="data of tasks in single trace", "folder name"=w196, "file name"=w169, "Processed data"=w183) -> (w193:T25)
              }
              n145 = flat-sequence "initialize list" {
                tunnel: w110 -> [w149]
                tunnel: w96 -> [w148]
                tunnel: [w148] -> w95
                frame #0 {
                  w150 = 0  # default trace
                  n146 = Index Array(array=w149, index=w150) -> (element=w155:T27)
                  n147 = for {
                    tunnel: w149 -> [w159] mode=indexing
                    tunnel: [w158] -> w156 mode=indexing
                    n148 = Unbundle(w159) -> ("trace name"=w158:string)  [unwired: 4 out]
                  }
                  n149 = Unbundle(w155) -> ("tasklist (name)"=w153:string[])  [unwired: 4 out]
                  n150 = control-ref of="All tasks in tasklist"() -> (w154:refnum<vi>)
                  n151 = control-ref of="All traces"() -> (w157:refnum<vi>)
                  n152 = property class="LstBox (strict)"(reference=w154, "Item Names"=w153) -> ()  [unwired: 1 in, 2 out]
                  n153 = property class="LstBox (strict)"(reference=w157, "Item Names"=w156) -> (reference out=w152:refnum<vi>, error out=w151:errorcluster)  [unwired: 1 in]
                  n154 = property class="LstBox (strict)"(reference=w152, error in=w151, "Value"=w150) -> ()  [unwired: 2 out]
                }
              }
              n155 = Unbundle(w95) -> (w99:T33, "trace name"=w104:string)  [unwired: 3 out]
              n156 = Concatenate Strings("Processed" ("string"), w104) -> (w102:string)
              n157 = Build Path(base path=w98, name or relative path=w102) -> (appended path=w108:path)
              n158 = call <vilib>:"Check if File or Folder Exists.vi"("path"=w108) -> ("error out"=w106:errorcluster, "file or folder exists?"=w101:bool, "dup path"=w107:path)  [unwired: 8 in]
              n159 = case shown="False" w101 {
                tunnel: w107 -> [w145 w147]
                tunnel: w106 -> [w144 w146]
                tunnel: [w143 w147] -> w105
                tunnel: [w142 w146] -> w100
                frame False {
                  n160 = Create Folder(path (use dialog)=w145, error in=w144) -> (created path=w143:path, error out=w142:errorcluster)  [unwired: 1 in, 1 out]
                }
                frame True {
                }
              }
              n161 = for {
                tunnel: w105 -> [w141]
                shift-right: [w139] -> _
                shift-left: w100 -> [w138]
                tunnel: w99 -> [w140] mode=indexing
                n162 = Unbundle(w140) -> ("task (file) name"=w135:string, "processed data"=w136:T24[])  [unwired: 1 out]
                n163 = Build Path(base path=w141, name or relative path=w135) -> (appended path=w137:path)
                n164 = call "SaveFlattenedData.vi"("error in (no error)"=w138, "Flattened data to be saved"=w136, "path in"=w137) -> ("error out"=w139:errorcluster)  [unwired: 3 in, 1 out]
              }
              n165 = Bundle(cluster=w112, w119, "tasklist (name)"=w118, "trace name"=w113, "description"=w117, "Array of Params"=w114) -> (w96:T27)
              n166 = case shown="True" FALSE {
                tunnel: [w131 w134] -> w111
                tunnel: w110 -> [w131 w133]
                tunnel: w96 -> [_ w132]
                frame False {
                }
                frame True {
                  n167 = Build Array (concatenate)(w133, w132) -> (w134:T23)
                  "~All data converted" <- w134
                }
              }
              "Trace #" <- w127
            }
          }
        }
        n168 = local write "Start conversion"(w25) -> ()
      }
      event "stop": Value Change {
        n169 = event-data() -> ()  [unwired: 1 in, 6 out]
      }
    }
  }
  n170 = while {
    tunnel: w15 -> [_]
    tunnel: "Max digit of index" -> [w424]
    tunnel: "Key words" -> [w423]
    tunnel: w9 -> [w422]
    tunnel: w8 -> [w421]
    tunnel: w3 -> [w420]
    tunnel: w4 -> [_]
    stop <- w425 stop-if-true
    n171 = event shown="[9] \"Save graph\": Value Change" {
      selector: _ -> [_ _ _ _ _ _ _ _ _ _ _ _ _]
      dyn-events: _ -> [_ _ _ _ _ _ _ _ _ _ _ _ _]
      timeout: _ -> [_ _ _ _ _ _ _ _ _ _ _ _ _]
      tunnel: [_ _ _ _ w619 _ _ _ _ _ _ _ _] -> w425
      tunnel: w424 -> [w445 _ _ _ _ _ _ _ _ _ _ _ _]
      tunnel: w423 -> [w447 _ _ _ _ _ _ _ _ _ _ _ _]
      tunnel: w422 -> [_ _ _ _ _ _ _ _ _ _ _ _ _]
      tunnel: w421 -> [_ _ _ _ _ _ _ _ _ _ _ _ _]
      tunnel: w420 -> [_ _ _ _ _ _ _ _ _ _ _ _ _]
      event "Apply new \"config.ini\" file", "Raw data root folder", "configuration file path": Value Change {
        n172 = event-data() -> ()  [unwired: 1 in, 6 out]
        n173 = control-ref of="Warning message"() -> (w443:refnum<vi>)
        n174 = property on="key words in description" class="Str"() -> (error out=w436:errorcluster, "Value"=w437:string)  [unwired: 2 in, 1 out]
        n175 = property class="Str"(reference=w443, "Blinking"=FALSE, "Visible"=TRUE, "Value"="") -> (reference out=w440:refnum<vi>, error out=w441:errorcluster)  [unwired: 1 in]
        n176 = control-ref of="configuration file path"() -> (w433:refnum<vi>)
        n177 = call "AllFolderInfo.vi"("error in (no error)"=w441, "Root"="Raw data root folder", "Max digit of index"=w445, "Key words"=w447) -> ("error out"=w435:errorcluster, "Folder order correct? (Last mod : index)"=w448:bool, "data folder info"=w438:T35)  [unwired: 1 out]
        "All trace  info" <- w438
        n178 = property on="key words in description" class="Str"(error in=w436, "Val(Sgnl)"=w437) -> ()  [unwired: 1 in, 2 out]
        n179 = case shown="True" "Apply new \"config.ini\" file" {
          selector: "Apply new \"config.ini\" file" -> [_ w450]
          frame False {
          }
          frame True {
            n180 = property on="Recalculate params" class="Bool (strict)"("Val(Sgnl)"=w450) -> ()  [unwired: 2 in, 2 out]
          }
        }
        n181 = property class="Path"(reference=w433, "Visible"=TRUE) -> ()  [unwired: 1 in, 2 out]
        n182 = Not(x=w448) -> (.not. x?=w449:bool)
        n183 = property class="Str"(reference=w440, "Blinking"=w449, "Visible"=w449, "Value"="Inconsistency in folder modification date and index!") -> ()  [unwired: 1 in, 2 out]
        n184 = case shown="No Error" w435 {
          frame No Error {
          }
          frame Error {
          }
        }
        n185 = Index Array(array="empty data info") -> (element=w430:T28)  [unwired: 1 in]
        n186 = for {
          N -> [w455]
          tunnel: "Raw data root folder" -> [w470]
          tunnel: w445 -> [w482]
          tunnel: w438 -> [w481] mode=indexing
          shift-right: [w478] -> w429
          shift-left: "empty data info" -> [w464]
          tunnel: "configuration file path" -> [w463]
          tunnel: "Apply new \"config.ini\" file" -> [w457]
          tunnel: w430 -> [w451]
          i -> [w453]
          n187 = Unbundle By Name(w481) -> ("Folder name"=w469:string, "Folder index"=w475:i32, "Description"=w474:string)
          n188 = Empty String/Path?(string/path=w463) -> (empty?=w461:bool)
          n189 = Not A Number/Path/Refnum?(number/path/refnum=w463) -> (NaN/Path/Refnum?=w462:bool)
          n190 = Increment(x=w453) -> (x+1=w452:i32)
          n191 = call <vilib>:"Check if File or Folder Exists.vi"("path"=w463) -> ("file or folder exists?"=w460:bool)  [unwired: 8 in, 2 out]
          n192 = Divide(x=w452, y=w455) -> (x/y=→"pb1":dbl)
          n193 = Not(x=w461) -> (.not. x?=w458:bool)
          n194 = Not(x=w462) -> (.not. x?=w459:bool)
          n195 = Compound Arithmetic op=AND(w457, w460, w459, w458) -> (w456:bool)
          n196 = Build Path ("root of single trace (\"trace_000X\")")(base path=w470, name or relative path=w469) -> (appended path=w471:path)
          n197 = Build Path ("root of single trace (\"trace_000X\")")(base path=w470, name or relative path=w469) -> (appended path=w476:path)
          n198 = Build Path ("path of params")(base path=w471, name or relative path="DAQ.tasklist") -> (appended path=w472:path)
          n199 = Build Path ("path of params")(base path=w476, name or relative path="Params.bin") -> (appended path=w479:path)
          n200 = call <vilib>:"Check if File or Folder Exists.vi"("path"=w472) -> ("file or folder exists?"=w468:bool, "dup path"=w467:path)  [unwired: 8 in, 1 out]
          n201 = call <vilib>:"Check if File or Folder Exists.vi"("path"=w479) -> ("file or folder exists?"=w466:bool, "dup path"=w477:path)  [unwired: 8 in, 1 out]
          n202 = And(x=w466, y=w468) -> (x .and. y?=w465:bool)
          n203 = case shown="True" w465 {
            tunnel: w482 -> [_ w504]
            tunnel: w464 -> [w483 w486]
            tunnel: [w483 w498] -> w478
            tunnel: w477 -> [_ w499]
            tunnel: w463 -> [_ w495]
            tunnel: w456 -> [_ w493]
            tunnel: w475 -> [_ w487]
            tunnel: w474 -> [_ w490]
            tunnel: w467 -> [_ _]
            tunnel: w451 -> [_ w484]
            frame False {
            }
            frame True {
              w506 = 1 items=["Write", "Read"] ("write (0) or read (1)")
              n204 = Strip Path(path=w499) -> (stripped path=w496:path)  [unwired: 1 out]
              n205 = call "ParamsArray2BinFile.vi"("write (0) or read (1)"=w506, "file path in"=w499) -> ("Array of Params out"=w494:T3[])  [unwired: 6 in, 3 out]
              n206 = List Folder(path=w496) -> (path out=w501:path, filenames=w505:string[])  [unwired: 3 in, 2 out]
              n207 = case shown="True" w493 {
                tunnel: w495 -> [_ w510]
                tunnel: w494 -> [w507 w509]
                tunnel: [w507 w508] -> w485
                frame False {
                }
                frame True {
                  n208 = for {
                    tunnel: w509 -> [w514] mode=indexing
                    tunnel: w510 -> [w512]
                    tunnel: [w513] -> w508 mode=indexing
                    w511 = u16 0 items=["Read to cluster Params from ini files", "Write to ini file from cluster Params", "Copy ini file to new Path"] ("Ring")
                    n209 = call "Setup4 Config.vi"("Ring"=w511, "Config file to read/write"=w512, "Params in"=w514) -> ("Params out"=w513:T3)  [unwired: 6 in, 2 out]
                  }
                }
              }
              n210 = for {
                tunnel: w505 -> [w523] mode=indexing
                tunnel: w504 -> [w528]
                shift-right: [w527] -> w492
                shift-left: cluster{"Folder index":i32, path, string}[] [] -> [w525]
                tunnel: w501 -> [w524]
                n211 = Build Path(base path=w524, name or relative path=w523) -> (appended path=w521:path)
                n212 = case shown="False" TRUE {
                  tunnel: w528 -> [w532 w546]
                  tunnel: [w533 w543] -> w526
                  tunnel: w523 -> [w529 w540]
                  tunnel: [w534 w539] -> w522
                  tunnel: w521 -> [w537 w538]
                  frame False {
                    n213 = call <vilib>:"Get File Extension.vi"("file"=w537) -> ("lowercase file extension"=w536:string, "dup file"=w531:path)  [unwired: 6 in, 3 out]
                    n214 = call "Basci_VIs_FindIndexByKeyWords.vi"("Max length\nof index"=w532, "String input"=w529) -> ("Folder index"=w530:i32)  [unwired: 2 in, 3 out]
                    n215 = Bundle("Folder index"=w530, "dup file"=w531, w529) -> (w533:T36)  [unwired: 1 in]
                    n216 = Equal?(x="txt", y=w536) -> (x = y?=w534:bool)
                  }
                  frame True {
                    n217 = call "Basci_VIs_FindIndexByKeyWords.vi"("Max length\nof index"=w546, "Key words"="_", "String input"=w540) -> ("Log"=w544:string, "Folder index"=w541:i32)  [unwired: 1 in, 2 out]
                    n218 = Bundle("Folder index"=w541, "appended path"=w538, w540) -> (w543:T37)  [unwired: 1 in]
                    n219 = Not Equal?(x="No key words", y=w544) -> (x != y?=w539:bool)
                  }
                }
                n220 = case shown="True" w522 {
                  tunnel: [w547 w550] -> w527
                  tunnel: w526 -> [_ w549]
                  tunnel: w525 -> [w547 w548]
                  frame False {
                  }
                  frame True {
                    n221 = Build Array (concatenate)(w548, w549) -> (w550:T38)
                  }
                }
              }
              n222 = Array Size(array=w494) -> (size(s)=w500:i32)
              n223 = Sort 1D Array(array=w492) -> (sorted array=w491:cluster{"Folder index":i32, path, string}[])
              n224 = Array Size(array=w491) -> (size(s)=w502:i32)
              n225 = Not Equal?(x=w502, y=w500) -> (x != y?=w497:bool)
              n226 = case shown="True" w497 {
                frame False {
                }
                frame True {
                  w518 = TRUE ("Blinking")
                  n227 = local read "Warning message"() -> (w516:string)
                  n228 = control-ref of="Warning message"() -> (w519:refnum<vi>)
                  n229 = Concatenate Strings(w516, "Warning: one or multiple tasks are missing" ("Value")) -> (w517:string)
                  n230 = property class="Str"(reference=w519, "Blinking"=w518, "Visible"=w518, "Value"=w517) -> ()  [unwired: 1 in, 2 out]
                }
              }
              n231 = Bundle(cluster=w484, "trace#"=w487, w491, "description"=w490, "Convert?"=TRUE, "params array"=w485) -> (w489:T28)  [unwired: 1 in]
              n232 = Build Array (concatenate)(w486, w489) -> (w498:T2)
            }
          }
        }
        n233 = Reverse 1D Array(array=w429) -> (reversed array=w428:T2)
        n234 = local write "Data info"(w428) -> ()
      }
      event "refresh trace list": Value Change {
        n235 = event-data() -> ()  [unwired: 1 in, 6 out]
        n236 = control-ref of="All traces"() -> (w568:refnum<vi>)
        n237 = property class="LstBox (strict)"(reference=w568) -> (reference out=w567:refnum<vi>, "Value"=w565:i32, "Item Names"=w566:string[])  [unwired: 1 in, 1 out]
        n238 = Array Size(array=w566) -> (size(s)=w564:i32)
        n239 = local write "refresh trace list"(FALSE ("refresh trace list")) -> ()
        n240 = Decrement(x=w564) -> (x-1=w563:i32)
        n241 = local read "~All data converted"() -> (w560:T23)
        n242 = control-ref of="All tasks in tasklist"() -> (w562:refnum<vi>)
        n243 = Max & Min(x=w565, y=w563) -> (min(x,y)=w559:i32)  [unwired: 1 out]
        n244 = Max & Min(x=w559, y=0) -> (max(x,y)=w557:i32)  [unwired: 1 out]
        n245 = Index Array(array=w560, index=w557) -> (element=w553:T27)
        n246 = for {
          tunnel: w560 -> [w570] mode=indexing
          tunnel: [w569] -> w552 mode=indexing
          n247 = Unbundle(w570) -> ("trace name"=w569:string)  [unwired: 4 out]
        }
        n248 = Unbundle(w553) -> ("tasklist (name)"=w554:string[], "description"=w551:string)  [unwired: 3 out]
        n249 = local write "Description"(w551) -> ()
        n250 = property class="LstBox (strict)"(reference=w562, "Item Names"=w554) -> ()  [unwired: 1 in, 2 out]
        n251 = property class="LstBox (strict)"(reference=w567, "Item Names"=w552) -> (reference out=w555:refnum<vi>, error out=w556:errorcluster)  [unwired: 1 in]
        n252 = property class="LstBox (strict)"(reference=w555, error in=w556, "Val(Sgnl)"=w557) -> ()  [unwired: 2 out]
      }
      event "Delete trace", "Undo delete": Value Change {
        w588 = FALSE ("Undo delete")
        n253 = event-data() -> ()  [unwired: 1 in, 6 out]
        n254 = local read "array delete order"() -> (w583:i32[])
        n255 = local read "~All data converted"() -> (w572:T23)
        n256 = local write "Undo delete"(w588) -> ()
        n257 = local write "Delete trace"(w588) -> ()
        n258 = Array Size(array=w583) -> (size(s)=w582:i32)
        n259 = Array Size(array=w572) -> (size(s)=w577:i32)
        n260 = Not Equal?(x=0, y=w582) -> (x != y?=w580:bool)
        n261 = Not Equal?(x=w577, y=0 ("x")) -> (x != y?=w575:bool)
        n262 = And(x="Undo delete", y=w580) -> (x .and. y?=w578:bool)
        n263 = control-ref of="All traces"() -> ()  [unwired: 1 out]
        n264 = And(x=w575, y="Delete trace") -> (x .and. y?=w573:bool)
        n265 = control-ref of="refresh trace list"() -> (w590:refnum<vi>)
        n266 = case shown="True" w573 {
          tunnel: [_ w608] -> w589
          tunnel: w572 -> [_ w603]
          frame False {
          }
          frame True {
            n267 = control-ref of="All traces"() -> (w609:refnum<vi>)
            n268 = property class="LstBox (strict)"(reference=w609) -> (error out=w608:errorcluster, "Value"=w605:i32)  [unwired: 1 in, 1 out]
            n269 = local read "array delete order"() -> (w607:i32[])
            n270 = local read "data deleted"() -> (w612:T23)
            n271 = Delete From Array(array=w603, length=1, index=w605) -> (deleted portion=w611:T23, array with subset deleted=w604:T23)
            n272 = local write "~All data converted"(w604) -> ()
            n273 = Build Array (concatenate)(w611, w612) -> (→"data deleted":T23)
            n274 = Build Array (concatenate)(w605, w607) -> (→"array delete order":i32[])
          }
        }
        n275 = case shown="True" w578 {
          tunnel: w589 -> [_ _]
          tunnel: w583 -> [_ w592]
          frame False {
          }
          frame True {
            w598 = 0 ("index")
            w599 = 1 ("length")
            n276 = local read "data deleted"() -> (w602:T23)
            n277 = Delete From Array(array=w602, length=w599, index=w598) -> (deleted portion=w596:T23, array with subset deleted=w601:T23)
            n278 = Delete From Array(array=w592, length=w599, index=w598) -> (deleted portion=w594:i32[], array with subset deleted=w600:i32[])
            n279 = local write "array delete order"(w600) -> ()
            n280 = local write "data deleted"(w601) -> ()
            n281 = Index Array(array=w594) -> (element=w593:i32)  [unwired: 1 in]
            n282 = local read "~All data converted"() -> (w597:T23)
            n283 = Insert Into Array(array=w597, index=w593, new element=w596) -> (w595:T23)
            n284 = local write "~All data converted"(w595) -> ()
          }
        }
        n285 = property class="Bool (strict)"(reference=w590, "Val(Sgnl)"=TRUE ("Value (Signaling)")) -> (error out=w584:errorcluster)  [unwired: 1 in, 1 out]
        n286 = control-ref of="X Axis to plot"() -> (w571:refnum<vi>)
        n287 = property class="Ring (strict)"(reference=w571, error in=w584) -> (reference out=w587:refnum<vi>, error out=w585:errorcluster, "Value"=w586:i32)
        n288 = property class="Ring (strict)"(reference=w587, error in=w585, "Val(Sgnl)"=w586) -> ()  [unwired: 2 out]
      }
      event "Data Analysis Tab": Value Change {
        w616 = FALSE ("Blinking")
        n289 = event-data() -> ()  [unwired: 1 in, 6 out]
        n290 = control-ref of="Warning message"() -> (w615:refnum<vi>)
        n291 = property class="Str"(reference=w615, "Blinking"=w616, "Visible"=w616) -> ()  [unwired: 1 in, 2 out]
        n292 = case shown="\"Results\"" "Data Analysis Tab" {
          frame "Data conversion/Processed data import", Default {
          }
          frame "Results" {
            n293 = property on="All tasks in tasklist" class="LstBox (strict)"() -> (error out=w617:errorcluster, "Value"=w618:i32[])  [unwired: 2 in, 1 out]
            n294 = property on="All tasks in tasklist" class="LstBox (strict)"(error in=w617, "Val(Sgnl)"=w618) -> ()  [unwired: 1 in, 2 out]
          }
        }
      }
      event "stop": Value Change {
        n295 = event-data() -> ("NewVal"=w619:bool)  [unwired: 1 in, 5 out]
      }
      event "key words in description": Value Change; "key words in description": Key Down {
        n296 = event-data() -> ()  [unwired: 1 in, 4 out]
        n297 = call <vilib>:"Trim Whitespace.vi"("string"="key words in description") -> ("trimmed string"=w621:string)  [unwired: 1 in]
        n298 = local write "key words in description"(w621) -> ()
        n299 = local read "Data info"() -> (w622:T2)
        n300 = Array Size(array=w622) -> (size(s)=w623:i32)
        n301 = for {
          tunnel: [w640] -> w627 mode=indexing
          tunnel: w622 -> [w641] mode=indexing
          n302 = Unbundle(w641) -> ("description"=w640:string)  [unwired: 5 out]
        }
        n303 = for {
          N: w623 -> [_]
          shift-right: [w629] -> w624
          shift-left: w622 -> [w630]
          i -> [w628]
          n304 = in-place {
            n305 = in-place-array #1(w630, w628) -> (w632:T28)
            n306 = in-place {
              n307 = in-place-cluster #2(w632) -> ()  [unwired: 1 out]
              n308 = in-place-cluster #2("Convert?"=FALSE) -> (w631:T28)
            }
            n309 = in-place-array #1(w631) -> (w629:T2)  [unwired: 1 out]
          }
        }
        n310 = call "basic_subvi_and or search.vi"("key words"=w621, "String array input"=w627) -> ("index of string w/ key words"=w626:i32[])  [unwired: 2 in, 3 out]
        n311 = for {
          tunnel: w626 -> [w635] mode=indexing
          shift-right: [w634] -> w625
          shift-left: w624 -> [w636]
          n312 = in-place {
            n313 = in-place-array #3(w636, w635) -> (w638:T28)
            n314 = in-place {
              n315 = in-place-cluster #4(w638) -> ()  [unwired: 1 out]
              n316 = in-place-cluster #4("Convert?"=TRUE) -> (w637:T28)
            }
            n317 = in-place-array #3(w637) -> (w634:T2)  [unwired: 1 out]
          }
        }
        n318 = local write "Data info"(w625) -> ()
      }
      event "Y Axis to plot", "All traces", "All tasks in tasklist", "X Axis to plot": Value Change {
        w699 = 2.0 ("y")
        n319 = event-data() -> ()  [unwired: 1 in, 6 out]
        n320 = local read "~All data converted"() -> (w690:T23)
        n321 = control-ref of="All tasks in tasklist"() -> (w693:refnum<vi>)
        n322 = Index Array(array=w690, index="All traces") -> (element=w691:T27)
        n323 = Index Array(array="All tasks in tasklist") -> ()  [unwired: 1 in, 1 out]
        n324 = Unbundle(w691) -> (w694:T33, "tasklist (name)"=w692:string[], "description"=→"Description":string, "Array of Params"=→"Array of Params out":T3[])  [unwired: 1 out]
        n325 = for {
          tunnel: w694 -> [w783]
          tunnel: w693 -> [w781]
          tunnel: w692 -> [w780]
          tunnel: "All tasks in tasklist" -> [w779] mode=indexing
          tunnel: [w776] -> w676 mode=indexing
          tunnel: [w777] -> w650 mode=indexing
          tunnel: [w769] -> w675 mode=indexing
          tunnel: [w763] -> w653 mode=indexing
          tunnel: [w762] -> w652 mode=indexing
          w767 = 32 items=["V_A' [V]", "V_D' [V]", "V_P'  [V]", "V_S' [V]", "V_L' [V]", "V_R' [V]", "V_sum' [V]", "V_x [V]", "V_y [V]", "V_px' [V]", "V_py' [V]", "V_pz' [V]", "dt [s]", "Vpx_AO [V]", "Vpy_AO [V]", "Vpz_AO [V]", "scan backlog", "Counter", "TrapX [nm]", "TrapY [nm]", "TrapZ [nm]", "V_A [V]", "V_D [V]", "V_P [V]", "V_S [V]", "V_L [V]", "V_R [V]", "V_sum [V]", "V_x [V]", "V_y [V]", "P power [mW]", "S power [mW]", "angle compensated P power [W]", "angle compensated S power [W]", "angle compensated V_L", "angle compensated V_R", "angle compensated V_sum [V]", "angle compensated V_x [V]", "angle compensated V_y [V]", "Psi [rad]", "Laser power before objective[W]", "E_in", "E_out", "Delta E", "X signal", "Y signal", "Z signal", "TrapX (AO) [nm]", "TrapY (AO) [nm]", "TrapZ (AO) [nm]", "Fz [pN]", "Zext [nm]", "Tau [pNnm]", "Turn", "Fx [pN]", "Xext [nm]", "Fy [pN]", "Yext [nm]", "time [s]", "Delta Z signal", "Delta Z bead [nm]", "Z bead [nm]", "Delta TrapZ [nm]", "Delta Xsignal", "X bead [nm]", "Delta Ysignal", "Y bead [nm]", "Stop Condition"] ("Y Axis to plot 3")
          w768 = 33 items=["V_A' [V]", "V_D' [V]", "V_P'  [V]", "V_S' [V]", "V_L' [V]", "V_R' [V]", "V_sum' [V]", "V_x [V]", "V_y [V]", "V_px' [V]", "V_py' [V]", "V_pz' [V]", "dt [s]", "Vpx_AO [V]", "Vpy_AO [V]", "Vpz_AO [V]", "scan backlog", "Counter", "TrapX [nm]", "TrapY [nm]", "TrapZ [nm]", "V_A [V]", "V_D [V]", "V_P [V]", "V_S [V]", "V_L [V]", "V_R [V]", "V_sum [V]", "V_x [V]", "V_y [V]", "P power [mW]", "S power [mW]", "angle compensated P power [W]", "angle compensated S power [W]", "angle compensated V_L", "angle compensated V_R", "angle compensated V_sum [V]", "angle compensated V_x [V]", "angle compensated V_y [V]", "Psi [rad]", "Laser power before objective[W]", "E_in", "E_out", "Delta E", "X signal", "Y signal", "Z signal", "TrapX (AO) [nm]", "TrapY (AO) [nm]", "TrapZ (AO) [nm]", "Fz [pN]", "Zext [nm]", "Tau [pNnm]", "Turn", "Fx [pN]", "Xext [nm]", "Fy [pN]", "Yext [nm]", "time [s]", "Delta Z signal", "Delta Z bead [nm]", "Z bead [nm]", "Delta TrapZ [nm]", "Delta Xsignal", "X bead [nm]", "Delta Ysignal", "Y bead [nm]", "Stop Condition"] ("Y Axis to plot 3")
          n326 = property class="LstBox (strict)"(reference=w781, "Item Names"=w780) -> ()  [unwired: 1 in, 2 out]
          n327 = Index Array(array=w783, index=w779) -> (element=w782:T39)
          n328 = Unbundle(w782) -> ("processed data"=w775:T24[])  [unwired: 2 out]
          n329 = call "FlattenedData1Darray to 2Darray.vi"("Flattened data 1D array"=w775) -> ("2D array"=w774:dbl[][])  [unwired: 6 in]
          n330 = Index Array(array=w774, index (col) #1="X Axis to plot", index (col) #2="Y Axis to plot", index (col) #3=w767, index (col) #4="X Axis to plot 2", index (col) #5="Y Axis to plot 2", index (col) #6=w768) -> (element #1=w778:dbl[], element #2=w777:dbl[], element #3=w766:dbl[], element #4=w771:dbl[], element #5=w770:dbl[], element #6=w765:dbl[])  [unwired: 6 in]
          n331 = Add(x=w766, y=w765) -> (x+y=w764:dbl[])
          n332 = call <vilib>:"Std Deviation and Variance.vi"("X"=w764) -> ("mean"=w763:dbl, "standard deviation"=w762:dbl)  [unwired: 1 in, 1 out]
          n333 = Bundle("2D array"=w778, "2D array"=w777) -> (w776:cluster{"2D array":dbl[], "2D array":dbl[]})  [unwired: 1 in]
          n334 = Bundle("2D array"=w771, "2D array"=w770) -> (w769:cluster{"2D array":dbl[], "2D array":dbl[]})  [unwired: 1 in]
        }
        "XY Graph" <- w676
        "XY Graph for plot 1" <- w676
        "XY Graph for plot 2" <- w675
        n335 = control-ref of="Y Axis to plot 2"() -> (w654:refnum<vi>)
        n336 = control-ref of="Y Axis to plot"() -> (w655:refnum<vi>)
        n337 = control-ref of="X Axis to plot"() -> (w656:refnum<vi>)
        n338 = control-ref of="X Axis to plot 2"() -> (w657:refnum<vi>)
        n339 = control-ref of="X Axis to plot"() -> (w680:refnum<vi>)
        n340 = control-ref of="Y Axis to plot"() -> (w679:refnum<vi>)
        n341 = Build Array(w680, w679) -> (w689:refnum<vi>[])
        n342 = Build Array(w655, w654) -> (w658:refnum<vi>[])
        n343 = Build Array(w656, w657) -> (w659:refnum<vi>[])
        n344 = for "Auto name files based on displayed sections" {
          tunnel: w658 -> [w726] mode=indexing
          tunnel: w659 -> [w725] mode=indexing
          tunnel: [w724] -> w647 mode=indexing
          w734 = "_" ("string")
          n345 = control-ref of="All tasks in tasklist"() -> (w741:refnum<vi>)
          n346 = property class="LstBox (strict)"(reference=w741) -> ("Item Names"=w740:string[], "Value"=w739:i32[])  [unwired: 1 in, 2 out]
          n347 = property class="Ring (strict)"(reference=w726) -> ("Strings []"=w729:string[], "Value"=w728:i32)  [unwired: 1 in, 2 out]
          n348 = property class="Ring (strict)"(reference=w725) -> ("Strings []"=w732:string[], "Value"=w731:i32)  [unwired: 1 in, 2 out]
          n349 = for {
            tunnel: w740 -> [w752]
            tunnel: w739 -> [w751] mode=indexing
            shift-right: [w749] -> w737
            shift-left: "" -> [w750]
            n350 = Index Array(array=w752, index=w751) -> (element=w748:string)
            n351 = Search and Replace String(input string=w748, search string=".txt") -> (result string=w745:string)  [unwired: 6 in, 3 out]
            n352 = Concatenate Strings(w750, w745, "," ("string")) -> (w749:string)
          }
          n353 = Index Array(array=w729, index=w728) -> (element=w727:string)
          n354 = control-ref of="All traces"() -> (w744:refnum<vi>)
          n355 = Index Array(array=w732, index=w731) -> (element=w730:string)
          n356 = property class="LstBox (strict)"(reference=w744) -> ("Item Names"=w743:string[], "Value"=w742:i32)  [unwired: 1 in, 2 out]
          n357 = String Length(string=w737) -> (length=w736:i32)
          n358 = Decrement(x=w736) -> (x-1=w723:i32)
          n359 = String Subset(string=w737, length (rest)=w723) -> (substring=w735:string)  [unwired: 1 in]
          n360 = Index Array(array=w743, index=w742) -> (element=w720:string)
          n361 = Search and Replace String(input string=w720, search string="Processed") -> (result string=w721:string)  [unwired: 6 in, 3 out]
          n362 = Concatenate Strings(w721, w734, "Task_" ("string"), w735, w734, "Channels_" ("string"), w727, "_vs_" ("string"), w730) -> (w724:string)
        }
        n363 = for {
          tunnel: w689 -> [w804] mode=indexing
          tunnel: [w802] -> w688 mode=indexing
          n364 = property class="Ring (strict)"(reference=w804) -> ("Strings []"=w803:string[], "Value"=w801:i32)  [unwired: 1 in, 2 out]
          n365 = Index Array(array=w803, index=w801) -> (element=w802:string)
        }
        n366 = control-ref of="XY Graph"() -> (w706:refnum<vi>)
        n367 = control-ref of="Histogram Graph Y signal (the upmost task)"() -> (w682:refnum<vi>)
        n368 = call <vilib>:"Std Deviation and Variance.vi"("X"=w653) -> ("mean"=w646:dbl)  [unwired: 1 in, 2 out]
        "Laser power [W]" <- w646
        n369 = call <vilib>:"Std Deviation and Variance.vi"("X"=w652) -> ("mean"=→"Laser power fluctuation [W]":dbl)  [unwired: 1 in, 2 out]
        n370 = control-ref of="XY Graph"() -> (w665:refnum<vi>)
        n371 = control-ref of="XY Graph for plot 1"() -> (w666:refnum<vi>)
        n372 = Index Array(array=w688) -> (element #1=w687:string, element #2=w681:string)  [unwired: 2 in]
        n373 = for {
          tunnel: w650 -> [w717] mode=indexing
          shift-right: [w715] -> w648
          shift-left: dbl[] [] -> [w716]
          n374 = Build Array (concatenate)(w717, w716) -> (w715:dbl[])
        }
        n375 = property class="XYGraph (strict)"(reference=w682, "XScale.NameLbl.Text"=w681) -> ()  [unwired: 1 in, 2 out]
        n376 = Build Array(w666, w665) -> (w664:refnum<vi>[])
        n377 = for {
          tunnel: [w756] -> w695
          tunnel: w687 -> [w755]
          tunnel: w664 -> [w754] mode=indexing
          tunnel: w681 -> [w753]
          n378 = property on="Property Node" class="XYGraph (strict)"(reference=w754, "XScale.NameLbl.Text"=w755, "YScale.NameLbl.Text"=w753) -> (error out=w756:errorcluster)  [unwired: 1 in, 1 out]
        }
        n379 = property class="XYGraph (strict)"(reference=w706, error in=w695, "Active Cursor"=u32 0) -> (reference out=w708:refnum<vi>, error out=w709:errorcluster, "XScale.Maximum"=w704:dbl, "XScale.Minimum"=w705:dbl, "YScale.Maximum"=w701:dbl, "YScale.Minimum"=w700:dbl)
        n380 = Add(x=w701, y=w700) -> (x+y=w702:dbl)
        n381 = Add(x=w704, y=w705) -> (x+y=w703:dbl)
        n382 = Divide(x=w702, y=w699) -> (x/y=w697:dbl)
        n383 = Divide(x=w703, y=w699) -> (x/y=w698:dbl)
        n384 = Array Size(array=w648) -> (size(s)=w685:i32)
        n385 = Bundle(w698, w697) -> (w696:cluster{dbl, dbl})  [unwired: 1 in]
        n386 = control-ref of="X Axis to plot 2"() -> (w669:refnum<vi>)
        n387 = control-ref of="Y Axis to plot 2"() -> (w668:refnum<vi>)
        n388 = Greater?(x=w685, y=100) -> (0:w683:bool)
        n389 = property class="XYGraph (strict)"(reference=w708, error in=w709, "Cursor.Cursor Position"=w696) -> (reference out=w710:refnum<vi>, error out=w712:errorcluster)
        n390 = case shown="True" w683 {
          tunnel: w648 -> [_ w790]
          tunnel: w685 -> [_ w800]
          frame False {
          }
          frame True {
            n391 = Square Root(x=w800) -> (sqrt(x)=w799:dbl)
            n392 = Multiply(x=w799, y=0.2 ("x")) -> (x*y=w797:dbl)
            n393 = call <vilib>:"Std Deviation and Variance.vi"("X"=w790) -> ("mean"=→"mean":dbl, "standard deviation"=→"s.d.":dbl)  [unwired: 1 in, 1 out]
            n394 = call <vilib>:"Histogram.vi"("intervals"=w797, "X"=w790) -> ("Histogram Graph"=w792:T40)  [unwired: 6 in, 3 out]
            n395 = Unbundle(w792) -> ("X Values"=w794:dbl[], "Histogram: h(x)"=w796:i32[])
            n396 = call <vilib>:"Unconstrained Gaussian Peak Fit.vi"("Y"=w796, "X"=w794) -> ("Best Gaussian Fit"=w795:dbl[], "center"=→"center":dbl, "standard deviation"=→"sigma":dbl)  [unwired: 8 in, 3 out]
            n397 = Bundle("X Values"=w794, "Best Gaussian Fit"=w795) -> (w793:T41)  [unwired: 1 in]
            n398 = Build Array(w793, w792) -> (→"Histogram Graph Y signal (the upmost task)":T11)
          }
        }
        n399 = Build Array(w669, w668) -> (w673:refnum<vi>[])
        n400 = local read "Data (converted) to import"() -> (w662:path)
        n401 = property class="XYGraph (strict)"(reference=w710, error in=w712, "Active Cursor"=u32 1) -> (reference out=w713:refnum<vi>, error out=w714:errorcluster)
        n402 = property class="XYGraph (strict)"(reference=w713, error in=w714, "Cursor.Cursor Position"=w696) -> (error out=w667:errorcluster)  [unwired: 1 out]
        n403 = for {
          tunnel: w673 -> [w761] mode=indexing
          tunnel: [w759] -> w672 mode=indexing
          tunnel: w667 -> [w757]
          n404 = property class="Ring (strict)"(reference=w761, error in=w757) -> ("Strings []"=w760:string[], "Value"=w758:i32)  [unwired: 2 out]
          n405 = Index Array(array=w760, index=w758) -> (element=w759:string)
        }
        n406 = Index Array(array=w647) -> (element=w660:string)  [unwired: 1 in]
        n407 = local write "Graph autoname"(w647) -> ()
        n408 = Format Value(format string="_%.5f", value (0)=w646) -> (output string=w644:string)  [unwired: 1 in]
        n409 = Index Array(array=w672) -> (element #1=w671:string, element #2=w670:string)  [unwired: 2 in]
        n410 = control-ref of="XY Graph for plot 2"() -> (w674:refnum<vi>)
        n411 = Concatenate Strings(w660, w644, ".txt" ("string")) -> (w661:string)
        n412 = Build Path(base path=w662, name or relative path=w661) -> (appended path=w663:path)
        n413 = property on="Property Node" class="XYGraph (strict)"(reference=w674, "XScale.NameLbl.Text"=w671, "YScale.NameLbl.Text"=w670) -> ()  [unwired: 1 in, 2 out]
        n414 = local write "path"(w663) -> ()
      }
      event "save to txt": Value Change {
        n415 = event-data() -> ()  [unwired: 1 in, 6 out]
        n416 = case shown="True" "save to txt" {
          tunnel: [_ FALSE ("save to txt")] -> w805
          frame False {
          }
          frame True {
            w810 = dbl[] []
            n417 = local read "XY Graph"() -> (w811:T10)
            n418 = control-ref of="X Axis to plot"() -> (w817:refnum<vi>)
            n419 = control-ref of="Y Axis to plot"() -> (w822:refnum<vi>)
            n420 = for "Concatenate segments" {
              tunnel: w811 -> [w830] mode=indexing
              shift-right: [w825] -> w809
              shift-left: w810 -> [w827]
              shift-right: [w824] -> w808
              shift-left: w810 -> [w826]
              n421 = Unbundle(w830) -> ("Processed data"=w829:dbl[], "Processed data"=w828:dbl[])
              n422 = Build Array (concatenate)(w827, w829) -> (w825:dbl[])
              n423 = Build Array (concatenate)(w826, w828) -> (w824:dbl[])
            }
            n424 = property class="Ring (strict)"(reference=w817) -> ("Strings []"=w818:string[], "Value"=w819:i32)  [unwired: 1 in, 2 out]
            n425 = property class="Ring (strict)"(reference=w822) -> ("Strings []"=w820:string[], "Value"=w821:i32)  [unwired: 1 in, 2 out]
            n426 = Index Array(array=w818, index=w819) -> (element=w823:string)
            n427 = Index Array(array=w820, index=w821) -> (element=w814:string)
            n428 = Build Array(w823, w814) -> (w815:string[])
            n429 = Build Array(w809, w808) -> (w807:dbl[][])
            n430 = Transpose 2D Array(2D array=w807) -> (transposed array=w816:dbl[][])
            n431 = call "Save2DArrayWithColumnNames.vi"("2D data"=w816, "Column name array"=w815, "path in"="path") -> ()  [unwired: 7 in, 2 out]
          }
        }
        n432 = local write "save to txt"(w805) -> ()
      }
      event "Fit", "fit option": Value Change {
        n433 = event-data() -> ()  [unwired: 1 in, 6 out]
        n434 = case shown="True" "Fit" {
          tunnel: [_ FALSE ("Fit")] -> w831
          frame False {
          }
          frame True {
            n435 = control-ref of="XY Graph"() -> (w857:refnum<vi>)
            n436 = property class="XYGraph (strict)"(reference=w857) -> ("Value"=w874:T10)  [unwired: 1 in, 2 out]
            n437 = property class="XYGraph (strict)"(reference=w857, "Active Cursor"=u32 0) -> (reference out=w858:refnum<vi>, error out=w859:errorcluster)  [unwired: 1 in]
            n438 = for {
              tunnel: w874 -> [w882] mode=indexing
              shift-right: [w881] -> w846
              shift-left: dbl[] [] -> [w876]
              shift-right: [w880] -> w845
              shift-left: dbl[] [] -> [w877]
              n439 = Unbundle(w882) -> ("Processed data"=w879:dbl[], "Processed data"=w878:dbl[])
              n440 = Build Array (concatenate)(w876, w879) -> (w881:dbl[])
              n441 = Build Array (concatenate)(w877, w878) -> (w880:dbl[])
            }
            n442 = property class="XYGraph (strict)"(reference=w858, error in=w859) -> (reference out=w860:refnum<vi>, error out=w862:errorcluster, "Cursor.Cursor Position"=w865:T42)
            n443 = property class="XYGraph (strict)"(reference=w860, error in=w862, "Active Cursor"=u32 1) -> (reference out=w863:refnum<vi>, error out=w864:errorcluster)
            n444 = Build Cluster Array(w846, w845) -> (w873:cluster{"Force\n[pN]":dbl, "Force\n[pN]":dbl}[])
            n445 = Sort 1D Array(array=w873) -> (sorted array=w872:cluster{"Force\n[pN]":dbl, "Force\n[pN]":dbl}[])
            n446 = Unbundle(w865) -> ("Cursor X"=w869:dbl)  [unwired: 1 out]
            n447 = for {
              tunnel: w872 -> [w885] mode=indexing
              tunnel: [w884] -> w853 mode=indexing
              tunnel: [w883] -> w852 mode=indexing
              n448 = Unbundle(w885) -> ("Force\n[pN]"=w884:dbl, "Force\n[pN]"=w883:dbl)
            }
            n449 = property class="XYGraph (strict)"(reference=w863, error in=w864) -> (reference out=w836:refnum<vi>, error out=w835:errorcluster, "Cursor.Cursor Position"=w866:T42)
            n450 = Unbundle(w866) -> ("Cursor X"=w868:dbl)  [unwired: 1 out]
            n451 = Max & Min(x=w868, y=w869) -> (max(x,y)=w870:dbl, min(x,y)=w871:dbl)
            n452 = Threshold 1D Array(2:w870, 3:w853) -> (0:w856:dbl)  [unwired: 1 in]
            n453 = Threshold 1D Array(2:w871, 3:w853) -> (0:w855:dbl)  [unwired: 1 in]
            n454 = Subtract(x=w856, y=w855) -> (x-y=w854:dbl)
            n455 = Array Subset(array=w853, index=w855, length=w854) -> (w851:dbl[])
            n456 = Array Subset(array=w852, index=w855, length=w854) -> (w850:dbl[])
            n457 = case shown="2" "fit option" {
              tunnel: w851 -> [_ w893 w899 _]
              tunnel: w850 -> [_ w895 w900 _]
              tunnel: [T34 {"p"=0.0, "l0"=0.0, "k0"=0.0, "residue"=0.0} ("EWLC best fit parameters") w889 w897 T34 {"p"=0.0, "l0"=0.0, "k0"=0.0, "residue"=0.0} ("EWLC best fit parameters")] -> w849
              tunnel: [_ w887 w896 _] -> w837
              frame 0, Default {
              }
              frame 1 {
                w890 = 0.0
                n458 = call <vilib>:"Linear Fit.vi"("Y"=w895, "X"=w893) -> ("Best Linear Fit"=w894:dbl[], "slope"=w892:dbl, "intercept"=w891:dbl)  [unwired: 9 in, 2 out]
                n459 = Bundle(cluster=T9 {"coeff 0"=0.0, "coeff 1"=0.0, "coeff 2"=0.0, "coeff 3"=0.0}, "coeff 0"=w892, "coeff 1"=w891, "coeff 2"=w890, "coeff 3"=w890) -> (w889:T9)
                n460 = Bundle(w893, "Best Linear Fit"=w894) -> (w887:cluster{dbl[], "Best Linear Fit":dbl[]})  [unwired: 1 in]
              }
              frame 2 {
                n461 = call "EWLCfit.vi"("extension data"=w899, "force data"=w900) -> ("Force [pN] Extension [nm] output"=w898:cluster{"Y":dbl[], "X 2":dbl[]}[], "EWLC best fit parameters"=w897:T34)  [unwired: 5 in, 1 out]
                n462 = Index Array(array=w898) -> (element=w896:cluster{"Y":dbl[], "X 2":dbl[]})  [unwired: 1 in]
              }
              frame 3 {
              }
            }
            "Fitting result (see block diagram the meanings)" <- w849
            n463 = property class="XYGraph (strict)"(reference=w836, error in=w835) -> (reference out=w843:refnum<vi>, error out=w842:errorcluster, "Value"=w844:T10)
            n464 = property on="All tasks in tasklist" class="LstBox (strict)"() -> ("Value"=w839:i32[])  [unwired: 2 in, 2 out]
            n465 = Array Size(array=w839) -> (size(s)=w834:i32)
            n466 = Array Subset(array=w844, index=0, length=w834) -> (w841:T10)
            n467 = Build Array (concatenate)(w841, w837) -> (w840:cluster{"Y":dbl[], "X 2":dbl[]}[])
            n468 = property class="XYGraph (strict)"(reference=w843, error in=w842, "Value"=w840) -> ()  [unwired: 2 out]
          }
        }
        n469 = local write "Fit"(w831) -> ()
      }
      event "Save graph": Value Change {
        n470 = event-data() -> ("NewVal"=w903:bool)  [unwired: 1 in, 5 out]
        n471 = case shown="True" w903 {
          tunnel: [_ FALSE ("Save graph")] -> w904
          tunnel: [_ FALSE ("Save graph")] -> w902
          frame False {
          }
          frame True {
            n472 = local read "Data (converted) to import"() -> (w910:path)
            n473 = Unbundle By Name("Plot 1 Options") -> ("F: JPEG\nT: PNG"=w913:bool)
            n474 = Unbundle By Name("Plot 2 Options") -> ("F: JPEG\nT: PNG"=w912:bool)
            n475 = Build Array(w913, w912) -> (w911:bool[])
            n476 = for {
              tunnel: w911 -> [w935] mode=indexing
              tunnel: "Graph autoname" -> [w931] mode=indexing
              tunnel: w910 -> [w930]
              tunnel: [w932] -> w909 mode=indexing
              n477 = Path To String(path=w930) -> (string=w929:string)
              n478 = case shown="True" w935 {
                tunnel: [".JPG" ".PNG"] -> w934
                frame False {
                }
                frame True {
                }
              }
              n479 = String Length(string=w929) -> (length=w928:i32)
              n480 = Subtract(x=250 ("length (rest)"), y=w928) -> (x-y=w926:i32)
              n481 = String Subset(string=w931, length (rest)=w926) -> (substring=w925:string)  [unwired: 1 in]
              n482 = Concatenate Strings(w925, w934) -> (w933:string)
              n483 = Build Path(base path=w930, name or relative path=w933) -> (appended path=w932:path)
            }
            n484 = Index Array(array=w909) -> (element #1=w908:path, element #2=w907:path)  [unwired: 2 in]
            n485 = control-ref of="XY Graph for plot 2"() -> (w922:refnum<vi>)
            n486 = control-ref of="XY Graph for plot 1"() -> (w916:refnum<vi>)
            n487 = property on="Property Node" class="XYGraph (strict)"(reference=w916) -> ("XScale.NameLbl.Text"=w918:string, "YScale.NameLbl.Text"=w917:string)  [unwired: 1 in, 2 out]
            n488 = property on="Property Node" class="XYGraph (strict)"(reference=w922) -> ("XScale.NameLbl.Text"=w921:string, "YScale.NameLbl.Text"=w920:string)  [unwired: 1 in, 2 out]
            n489 = Bundle By Name(cluster="Plot 1 Options", "X axis label"=w918, "Y axis label"=w917) -> (w915:T14)
            n490 = Bundle By Name(cluster="Plot 2 Options", "X axis label"=w921, "Y axis label"=w920) -> (w919:T14)
            n491 = call "basic_subvi_plotPNG_v2_170407.vi"("Plot and Save Options"=w915, "Path"=w908, "Graph ref in"=w916) -> ()  [unwired: 8 in, 1 out]
            n492 = call "basic_subvi_plotPNG_v2_170407.vi"("Plot and Save Options"=w919, "Path"=w907, "Graph ref in"=w922) -> ()  [unwired: 8 in, 1 out]
          }
        }
        n493 = local write "Save graph"(w902) -> ()
        n494 = local write "Save graph"(w904) -> ()
      }
      event "Import converted data": Value Change {
        n495 = event-data() -> ("NewVal"=w950:bool)  [unwired: 1 in, 5 out]
        n496 = Empty String/Path?(string/path="Data (converted) to import") -> (empty?=w943:bool)
        n497 = Not A Number/Path/Refnum?(number/path/refnum="Data (converted) to import") -> (NaN/Path/Refnum?=w944:bool)
        n498 = Two Button Dialog(message="Import converted data will release all unsaved data in memory, continue?" ("消息"), 1:"Cancel" ("F按钮名称（“取消”）"), 2:"Continue" ("T按钮名称（“确定”）")) -> (T button?=w948:bool)
        n499 = call <vilib>:"Check if File or Folder Exists.vi"("path"="Data (converted) to import") -> ("file or folder exists?"=w939:bool)  [unwired: 8 in, 2 out]
        n500 = Not(x=w943) -> (.not. x?=w941:bool)
        n501 = Not(x=w944) -> (.not. x?=w940:bool)
        n502 = And(x=w950, y=w948) -> (x .and. y?=w949:bool)
        n503 = Compound Arithmetic op=AND(w941, w940, w939) -> (w938:bool)
        n504 = case shown="True" w938 {
          tunnel: [_ w960] -> w951
          tunnel: w949 -> [_ w959]
          tunnel: "Data (converted) to import" -> [_ w958]
          frame False {
            n505 = Two Button Dialog(message="Invalide data path" ("消息"), 1:"Cancel" ("F按钮名称（“取消”）"), 2:"Continue" ("T按钮名称（“确定”）")) -> ()  [unwired: 1 out]
          }
          frame True {
            n506 = case shown="False" "get description from raw data folder?" {
              tunnel: w958 -> [w970 w990]
              tunnel: [w964 w984] -> w957
              tunnel: [w961 w983] -> w956
              frame False {
                n507 = Build Path(base path=w970, name or relative path="AllDesc.txt") -> (appended path=w967:path)
                n508 = Open/Create/Replace File(file path (use dialog)=w967, operation (0:open)=T26."open or create", access (0:read/write)=enum16{"read/write", "read-only", "write-only"}."read-only") -> (refnum out=w965:refnum<file>, error out=w966:errorcluster)  [unwired: 3 in, 1 out]
                n509 = Read from Text File(file (use dialog)=w965, error in=w966) -> (text=w964:string)  [unwired: 2 in, 3 out]
                n510 = while {
                  tunnel: w964 -> [w981]
                  tunnel: [w973] -> w962 mode=indexing
                  tunnel: [w972] -> w963 mode=indexing
                  i -> [w982]
                  stop <- w979 stop-if-true
                  n511 = Pick Line(multi-line string=w981, line index=w982) -> (output string=w978:string)  [unwired: 1 in]
                  n512 = Equal?(x=w978, y="") -> (x = y?=w979:bool)
                  n513 = Search/Split String(string=w978, search string/char (-)="\t") -> (substring before match=w976:string, match + rest of string=w975:string)  [unwired: 1 in, 1 out]
                  n514 = String Subset(string=w975, offset (0)=1) -> (substring=w973:string)  [unwired: 1 in]
                  n515 = Decimal String To Number(string=w976) -> (number=w972:i32)  [unwired: 2 in, 1 out]
                }
                n516 = Bundle(w963, w962) -> (w961:cluster{i32[], string[]})  [unwired: 1 in]
              }
              frame True {
                n517 = Strip Path(path=w990) -> (stripped path=w987:path, name=w989:string)
                n518 = Search and Replace String(input string=w989, search string="_Processed") -> (result string=w986:string)  [unwired: 6 in, 3 out]
                n519 = Build Path(base path=w987, name or relative path=w986) -> (appended path=w985:path)
                n520 = call "Get all descriptions in project.vi"("Folder Path"=w985) -> ("All descriptions"=w984:string, "Descriptions and trace index"=w983:cluster{i32[], string[]})  [unwired: 7 in]
              }
            }
            "All descriptions" <- w957
            n521 = case shown="True" w959 {
              tunnel: [_ FALSE ("Import converted data")] -> w960
              tunnel: w958 -> [_ w1010]
              tunnel: w956 -> [_ w992]
              frame False {
              }
              frame True {
                n522 = List Folder(path=w1010) -> (path out=w1009:path, folder names=w1008:string[], error out=w1003:errorcluster)  [unwired: 3 in, 1 out]
                n523 = control-ref of="Importing traces.."() -> (w991:refnum<vi>)
                n524 = Array Size(array=w1008) -> (size(s)=w1007:i32)
                n525 = Decrement(x=w1007) -> (x-1=w1006:i32)
                n526 = property on="属性节点" class="Slide (strict)"(reference=w991, error in=w1003, "Scale.Maximum"=w1006, "Scale.Minimum"=0.0 ("Scale.Range:Minimum"), "Value"=-1) -> (error out=w1002:errorcluster)  [unwired: 1 out]
                n527 = for {
                  tunnel: w1008 -> [w1020] mode=indexing
                  tunnel: w1009 -> [w1041]
                  shift-right: [w1037] -> _
                  shift-left: w1002 -> [w1039]
                  tunnel: [w1025] -> w993 mode=indexing
                  tunnel: w992 -> [w1021]
                  i -> [w1015]
                  n528 = local read "Max digit of index"() -> (w1023:i32)
                  n529 = Build Path(base path=w1041, name or relative path=w1020) -> (appended path=w1040:path)
                  n530 = local read "Key words"() -> (w1022:string)
                  n531 = List Folder(path=w1040, error in=w1039) -> (path out=w1038:path, filenames=w1030:string[], error out=w1032:errorcluster)  [unwired: 2 in, 1 out]
                  n532 = Array Size(array=w1030) -> (size(s)=w1033:i32)
                  n533 = control-ref of="Task #"() -> (w1029:refnum<vi>)
                  n534 = Decrement(x=w1033) -> (x-1=w1034:i32)
                  n535 = property on="属性节点" class="Slide (strict)"(reference=w1029, error in=w1032, "Scale.Maximum"=w1034, "Scale.Minimum"=0.0 ("Scale.Range:Minimum"), "Value"=-1) -> (error out=w1031:errorcluster)  [unwired: 1 out]
                  n536 = Unbundle(w1021) -> (w1019:i32[], w1014:string[])
                  n537 = call "Basci_VIs_FindIndexByKeyWords.vi"("Max length\nof index"=w1023, "Key words"=w1022, "String input"=w1020) -> ("Folder index"=w1018:i32)  [unwired: 1 in, 3 out]
                  n538 = for {
                    tunnel: w1038 -> [w1062]
                    tunnel: w1030 -> [w1056] mode=indexing
                    shift-right: [w1059] -> w1037
                    shift-left: w1031 -> [w1060]
                    tunnel: [w1058] -> w1028 mode=indexing
                    tunnel: w1020 -> [w1055]
                    tunnel: [w1056] -> w1027 mode=indexing
                    tunnel: [w1055] -> w1026
                    i -> [w1057]
                    n539 = Build Path(base path=w1062, name or relative path=w1056) -> (appended path=w1061:path)
                    n540 = local write "Task #"(w1057) -> ()
                    n541 = call "BASIC_SUBVI_LoadDataWithColumnName.vi"("error in (no error)"=w1060, "path in"=w1061) -> ("error out"=w1059:errorcluster, "2D data"=w1054:dbl[][])  [unwired: 2 in, 2 out]
                    n542 = call "2Darray to FlattenedData1Darray.vi"("2D array"=w1054) -> ("Flattened data 1D array"=w1053:T24[])  [unwired: 6 in]
                    n543 = Bundle(w1055, w1056, "Flattened data 1D array"=w1053) -> (w1058:T43)  [unwired: 1 in]
                  }
                  n544 = for {
                    tunnel: w1019 -> [w1048] mode=indexing
                    tunnel: w1018 -> [w1046]
                    tunnel: w1014 -> [w1047]
                    shift-right: [w1045] -> w1016
                    shift-left: "" -> [w1044]
                    tunnel: [w1042] -> _ mode=indexing
                    i -> [w1043]
                    n545 = Equal?(x=w1048, y=w1046) -> (x = y?=w1042:bool)
                    n546 = case shown="True" w1042 {
                      tunnel: w1047 -> [_ w1052]
                      tunnel: w1043 -> [_ w1051]
                      tunnel: [w1049 w1050] -> w1045
                      tunnel: w1044 -> [w1049 _]
                      frame False {
                      }
                      frame True {
                        n547 = Index Array(array=w1052, index=w1051) -> (element=w1050:string)
                      }
                    }
                  }
                  n548 = local write "Description"(w1016) -> ()
                  n549 = Bundle(w1028, w1027, w1026, w1016, "Array of Params const"="Array of Params const") -> (w1025:T44)  [unwired: 1 in]
                  "Importing traces.." <- w1015
                }
                n550 = Index Array(array=w993) -> (element=w998:T44)  [unwired: 1 in]
                n551 = for {
                  tunnel: w993 -> [w1013] mode=indexing
                  tunnel: [w1012] -> w997 mode=indexing
                  n552 = Unbundle(w1013) -> (w1012:string)  [unwired: 4 out]
                }
                n553 = control-ref of="All tasks in tasklist"() -> (w999:refnum<vi>)
                n554 = control-ref of="All traces"() -> (w996:refnum<vi>)
                n555 = Unbundle(w998) -> (w1000:string[])  [unwired: 4 out]
                n556 = property class="LstBox (strict)"(reference=w996, "Item Names"=w997) -> (reference out=w994:refnum<vi>, error out=w995:errorcluster)  [unwired: 1 in]
                n557 = property class="LstBox (strict)"(reference=w999, "Item Names"=w1000) -> ()  [unwired: 1 in, 2 out]
                n558 = property class="LstBox (strict)"(reference=w994, error in=w995, "Val(Sgnl)"=0 ("值(信号)")) -> ()  [unwired: 2 out]
                n559 = local write "~All data converted"(w993) -> ()
              }
            }
          }
        }
        n560 = local write "Import converted data"(w951) -> ()
      }
      event "Data (converted) to import": Value Change {
        w1066 = 0.0 ("标尺.范围:最小值")
        w1065 = 0.0 ("标尺.范围:最小值")
        w1064 = 0 ("Value")
        n561 = event-data() -> ()  [unwired: 1 in, 6 out]
        n562 = control-ref of="Trace #"() -> (w1063:refnum<vi>)
        n563 = property class="Slide (strict)"(reference=w1063, "Value"=w1064) -> ()  [unwired: 1 in, 2 out]
        n564 = property class="Slide (strict)"(reference=w1063, "Value"=w1064) -> ()  [unwired: 1 in, 2 out]
        n565 = property on="属性节点" class="Slide (strict)"(reference=w1063, "Scale.Maximum"=w1065, "Scale.Minimum"=w1065) -> ()  [unwired: 1 in, 2 out]
        n566 = property on="属性节点" class="Slide (strict)"(reference=w1063, "Scale.Maximum"=w1066, "Scale.Minimum"=w1066) -> ()  [unwired: 1 in, 2 out]
      }
      event "CreateReport": Value Change {
        n567 = event-data() -> ("NewVal"=w1068:bool)  [unwired: 1 in, 5 out]
        n568 = case shown="True" w1068 {
          tunnel: [_ FALSE ("CreateReport")] -> w1067
          frame False {
          }
          frame True {
            n569 = local read "Data (converted) to import"() -> (w1072:path)
            n570 = call <vilib>:"New Report.vi"("report type"=enum16{"Standard Report", "HTML"}."Standard Report") -> ("report out"=w1074:refnum<class "NI_report.lvclass">, "error out"=w1073:errorcluster)  [unwired: 13 in]
            n571 = Build Path(base path=w1072, name or relative path="Report") -> (appended path=w1070:path)
            n572 = call-dynamic "Save Report to File.vi"("report in"=w1074, "report file path"=w1070, "prompt to replace? (F)"=TRUE ("Prompt to Replace? (F)"), "error in (no error)"=w1073) -> ()  [unwired: 10 in, 2 out]
          }
        }
        n573 = local write "CreateReport"(w1067) -> ()
      }
    }
  }
